vi "Wind_Turbine.vi"() -> (5 "Plug in titles":string[](array[string]), 7 "Plug in values":string[](array[string]))   [LabVIEW 2021]
uses:
  ADAM Client/Sub VIs/ADAM Controls/Channel_names.ctl
  <vilib>/Analysis/baseanly.llb/Mean (DBL).vi
  Globals/Meas_global.vi
  Globals/LDA_meas_global_1.vi
  <vilib>/Analysis/NI_AALBase.lvlib
  <vilib>/Analysis/NI_AALPro.lvlib
panel:
  in  "Time Shift":dbl
  out "X array":dbl[](array[numeric])
  out "WT Numbers":string[](array[string])
  out "WT Revolution Start times":dbl[](array[numeric])
  out "Laser Disp Index":i32
  out "Laser Phase lock index":i32
  out "Laser Status Index":i32
  out "L Status Phase lock index":i32
  in  "Tab Control":T1(tab)
  in  "Change Dem Voltages?":bool=TRUE
  in  "Allow large changes?":bool
  out "Turbine RPMs":cluster{i32[], "All WTs":dbl[]}(graph)
  out "All WTs":dbl[][](array[numeric]) format="%#.2g"
  out "Turbine Dem RPM":dbl[](array[numeric])
  out "Turbine Dem Voltage":dbl[](array[numeric])
  out "Cross Chs":cluster{dbl[], dbl[]}[](graph)
  in  "Cross_Corr to Phase Lock":i32[](listbox)
  in  "Channel to Phase lock":i32[](listbox)
  in  "Turbine to Phase Lock to":u16(ring) items=["RV (Ph)"]
  out "Inst Channels":cluster{dbl[], dbl[]}[](graph)
  in  "Add Phase data to results file":bool
  in  "Save Phase averaged Profiles":bool
  in  "Output Directory":path
  in  "Separation Character":string="\t"
  in  "Angular Step(deg)":dbl=1.0
  in  "Precision":string
  out "Av Disp 1":dbl
  out "Av Disp 2":dbl
  out "Av Disp 3":dbl
  out "Av Variance 1":dbl
  out "Av Variance 2":dbl
  out "Av Variance 3":dbl
  out "Angle 1":dbl format="%#_3g"
  out "Angle 2":dbl format="%#_3g"
  out "Angle 3":dbl format="%#_3g"
  out "Mean Blade 1":cluster{dbl, "Angular Step":dbl, dbl[]}(graph)
  out "slope 1":dbl format="%#_3g"
  out "Mean Blade 2":cluster{dbl, "Angular Step":dbl, dbl[]}(graph)
  out "Mean Blade 3":cluster{dbl, "Angular Step":dbl, dbl[]}(graph)
  out "slope 2":dbl format="%#_3g"
  out "slope 3":dbl format="%#_3g"
  out "Blade Positions":dbl[][](graph)
  out "Blade Angles":dbl[][](graph)
  out "Blade 1 Every Pass":dbl[](graph)
  out "Blade 2 Every Pass":dbl[](graph)
  out "Blade 3 Every Pass":dbl[](graph)
  out "Blade Analysis":string[][](table)
  in  "End Cut Deg":dbl
  in  "Start Cut Deg":dbl
  # "ADAM Channels"
  # "Rig_Name:Turbine_1:Dem_RPM"
  # "Rig_Name:Turbine_1:Dem_Volts"
  # "Mean RPM      SD RPM           Max-Min"
  # "Photo Darlington channel must have this symbol\nRV (Ph"
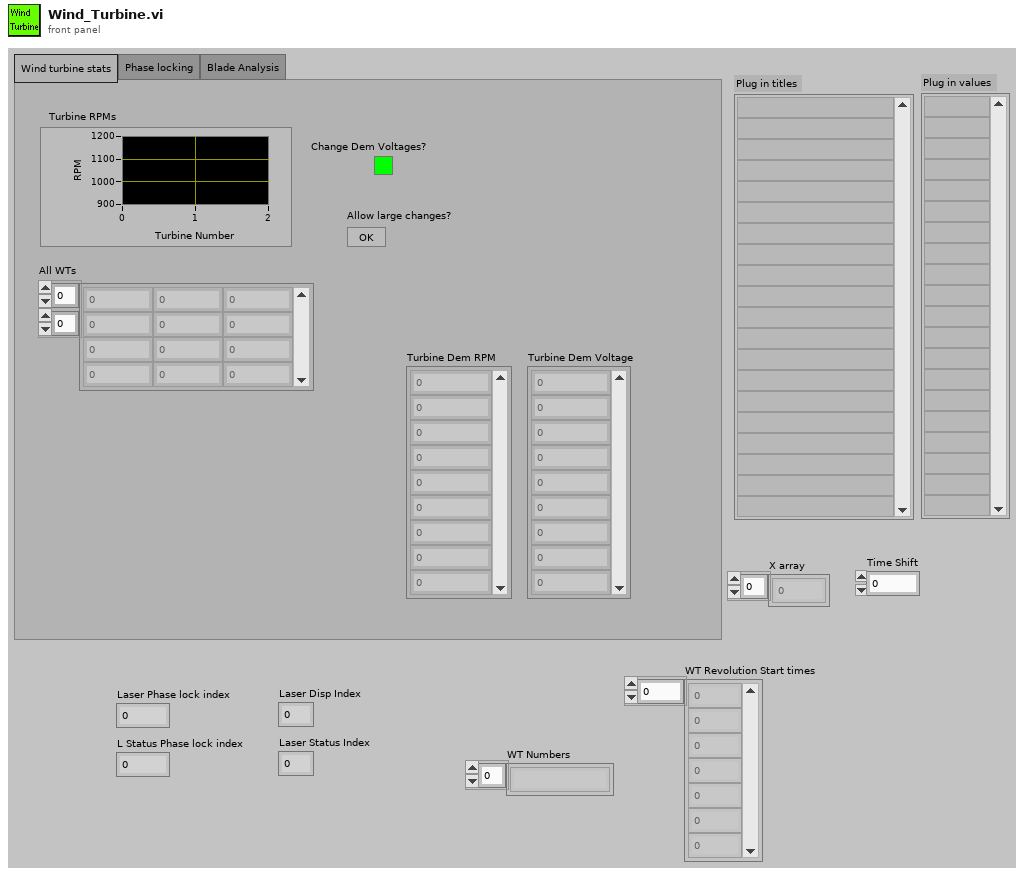
[diagram p1: front panel]
types:
  T1 = enum32{"Wind turbine stats", "Phase locking", "Blade Analysis"}
  T2 = typedef "Post_Process.ctl" = enum16{"Take New Data", "Post Process Raw Data File"}
  T3 = typedef "Analysis_info_cluster.ctl" = cluster{"Colour":u32, "Inst type":T4, "Inst name":string, "Symbol":string, "Code name":string, "Extra Info":string, "Inst Array":T5, "Extra Titles":string[], "Extra Values":string[], "U":dbl, "u^2":dbl, "u^3":dbl, "u^4":dbl, "Skew_u":dbl, "Kurt_u":dbl, "Sd Error in Mean":dbl, "% u'/U":dbl, "X":dbl, "Y":dbl, "Z":dbl, "Timescale integral Estimate":dbl, "Sd Error in Variance":dbl, "Calib File":path, "Calib Constants":dbl[], "Output Position":bool, "Stats":enum16{"None", "Basic", "Full"}, "Av Sampling Rate":dbl, "Av No of Samples":dbl, "Total Meas Time (s)":dbl, "ADAM Ch Name":string, "Max value":dbl, "Min value":dbl, "Req Sample Rate Hz":dbl, "Sync Delay Time (s)":dbl, "Ch No":i16, "Device":string, "Use Latest Calib":bool, "Port":string, "Metadata Ch Names":string[], "Metadata Ch Values":string[], "Label":string}
  T4 = typedef "Inst_type.ctl" = enum16{"Raw voltage", "Raw with zero offsetting", "Propeller anemometer", "Pressure Transducer", "Pitot-static tube", "Hot wire", "Cross wire 1", "Cross wire 2", "Generic Linear", "Generic Polynomial", "Generic BackPoly", "Fast FID", "Thermocouple", "Cold wire", "Pulsed Wire", "LDA Vel", "LDA Tran time", "LDA Arr time", "Microphone"}
  T5 = typedef "Instrument_Array.ctl" = enum16{"PWA", "LDA", "Analogue"}
  T6 = typedef "Time_Trace_Cluster.ctl" = cluster{"Weighting":dbl[], "Voltage":dbl[], "Eng Values":dbl[]}
  T7 = typedef "Channel_names.ctl" = enum16{"Active Only", "Active + Off", "All Channels", "Changeable Only"}
  T8 = typedef "Shift_Cluster.ctl" = cluster{"Stats":dbl[], "Spectra_Auto":dbl[], "Histogram":dbl[], "Hist Max":dbl, "Hist Min":dbl, "No of Samples":i32, "No in plume":i32, "Weight sum":dbl, "No Of Hist bins":i32, "TimeTrace Max":dbl, "Time Trace Min":dbl, "Trace St Deviation":dbl}
  T9 = typedef "Cross_Moments_Shift_Cluster.ctl" = cluster{"Stats":dbl[], "Resampled No of Samples":i32, "Resampled delta T":dbl, "Cross Correlation":dbl[]}
  T10 = cluster{"X array":dbl[], "Phase locked uw/u'w'":dbl[]}
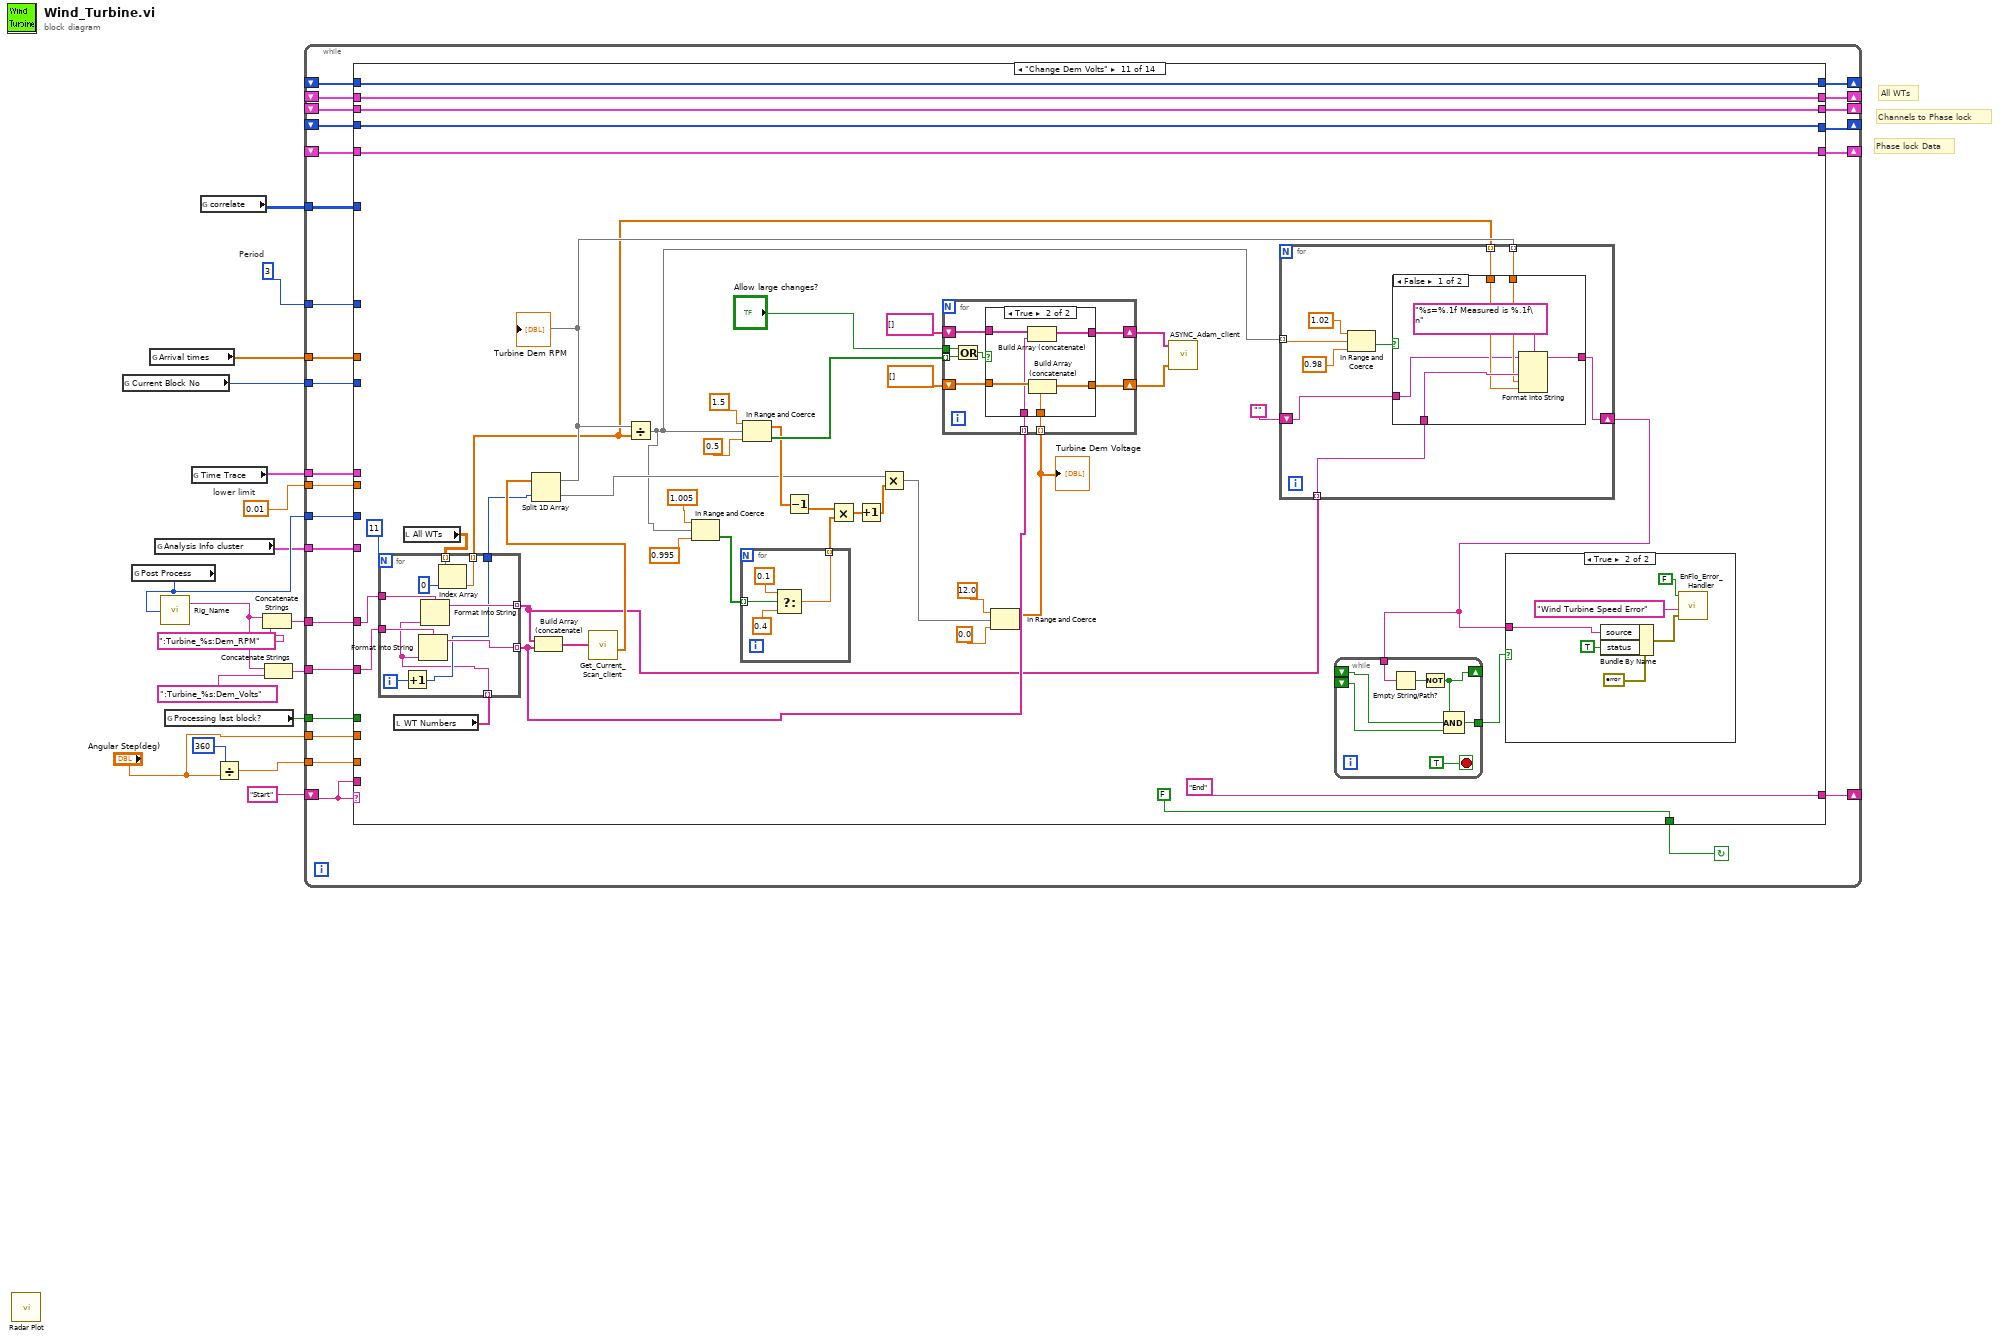
[diagram p0: block diagram]
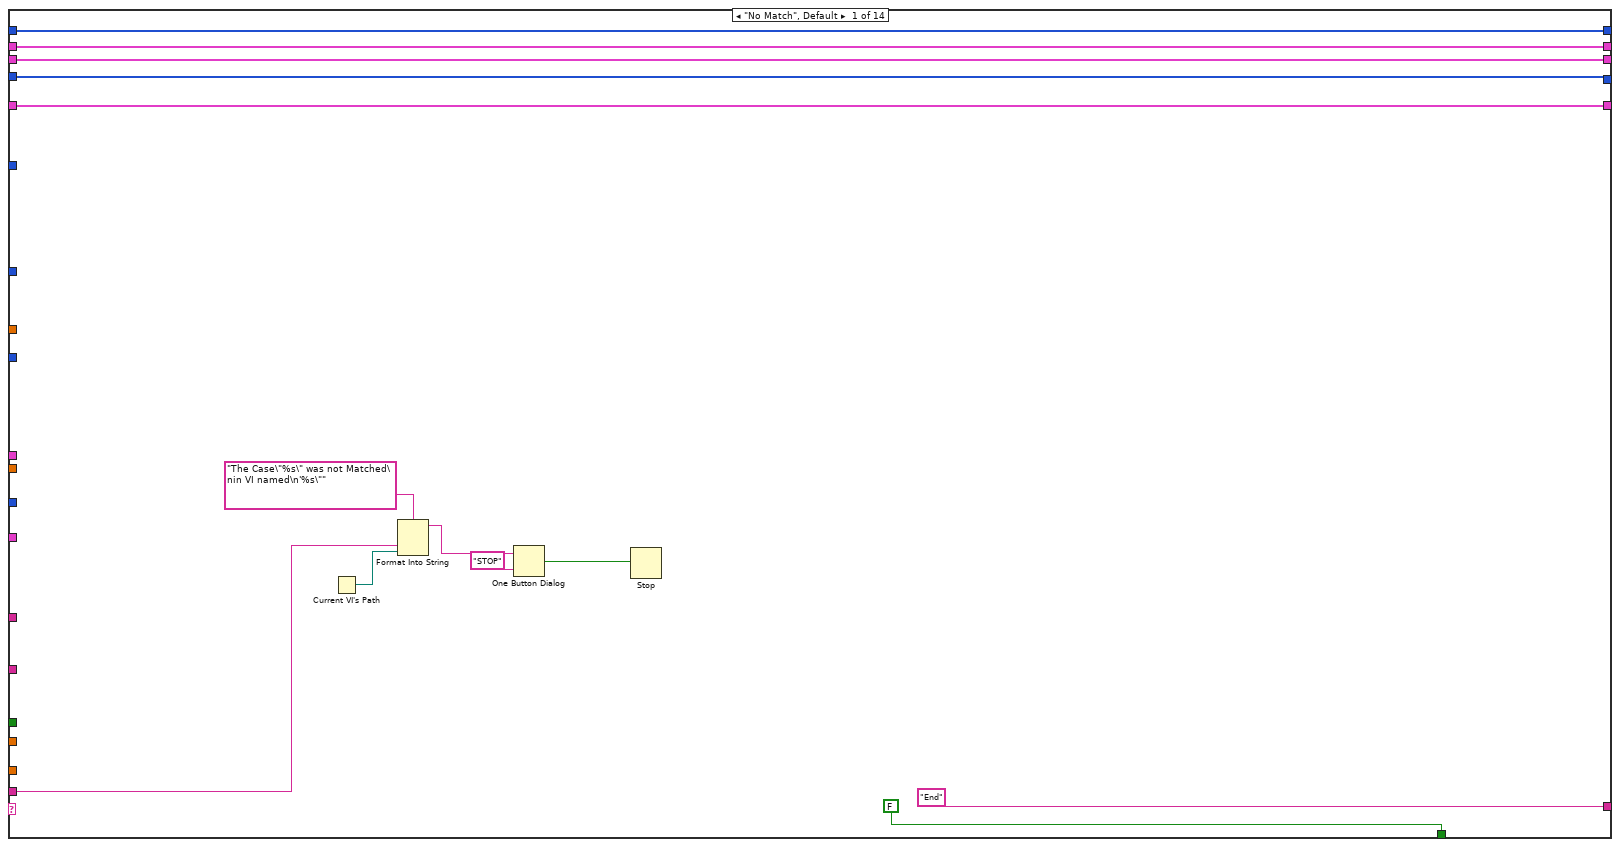
[diagram p2: hidden frame]
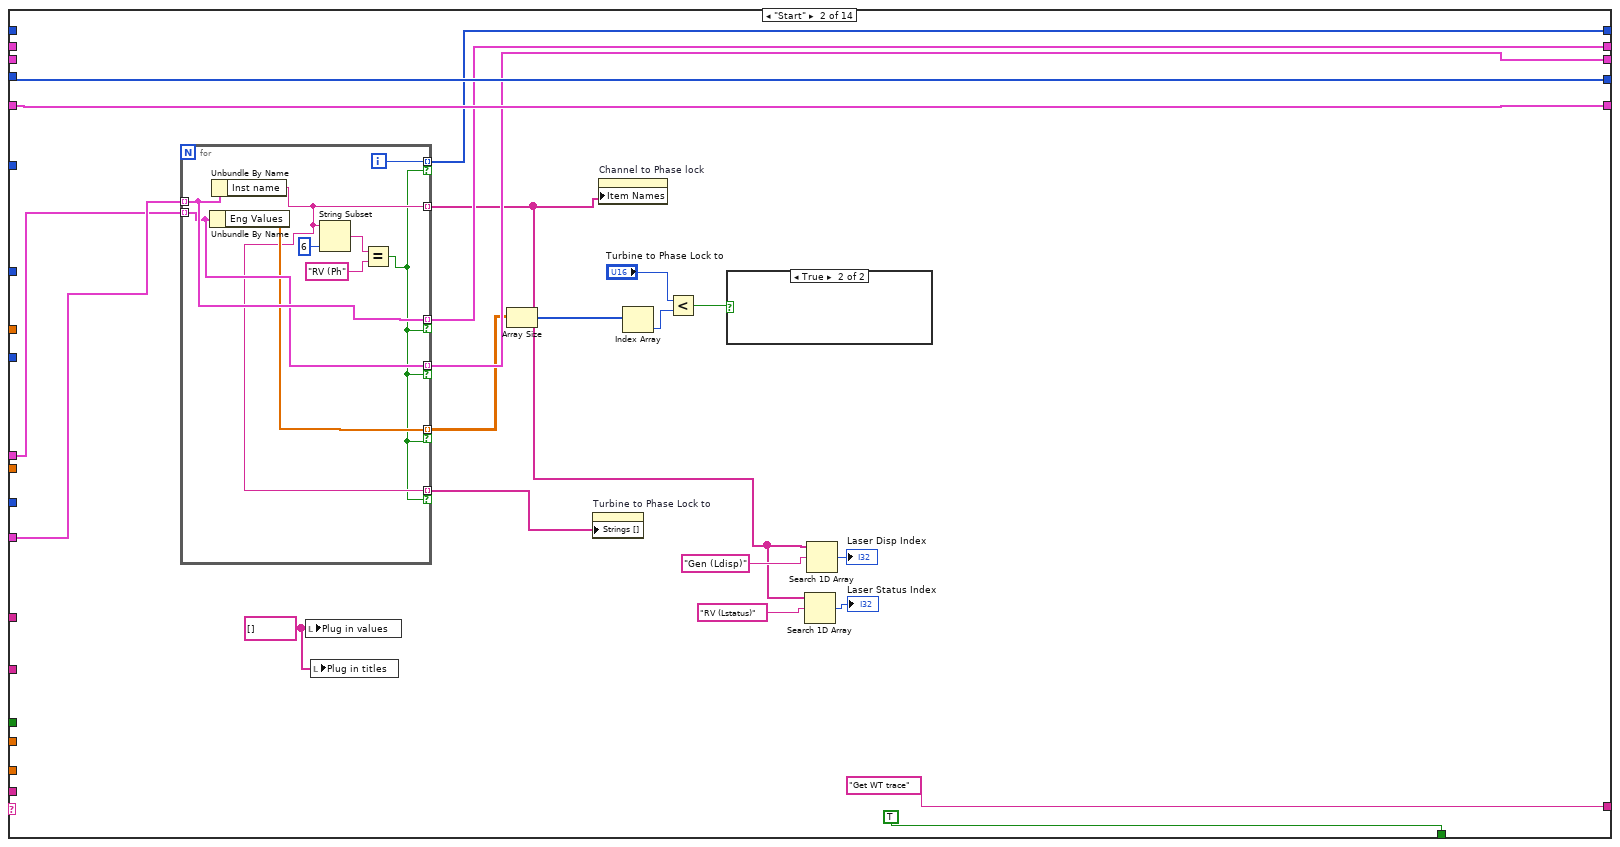
[diagram p3: hidden frame]
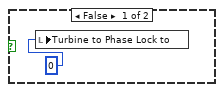
[diagram p4: hidden frame]
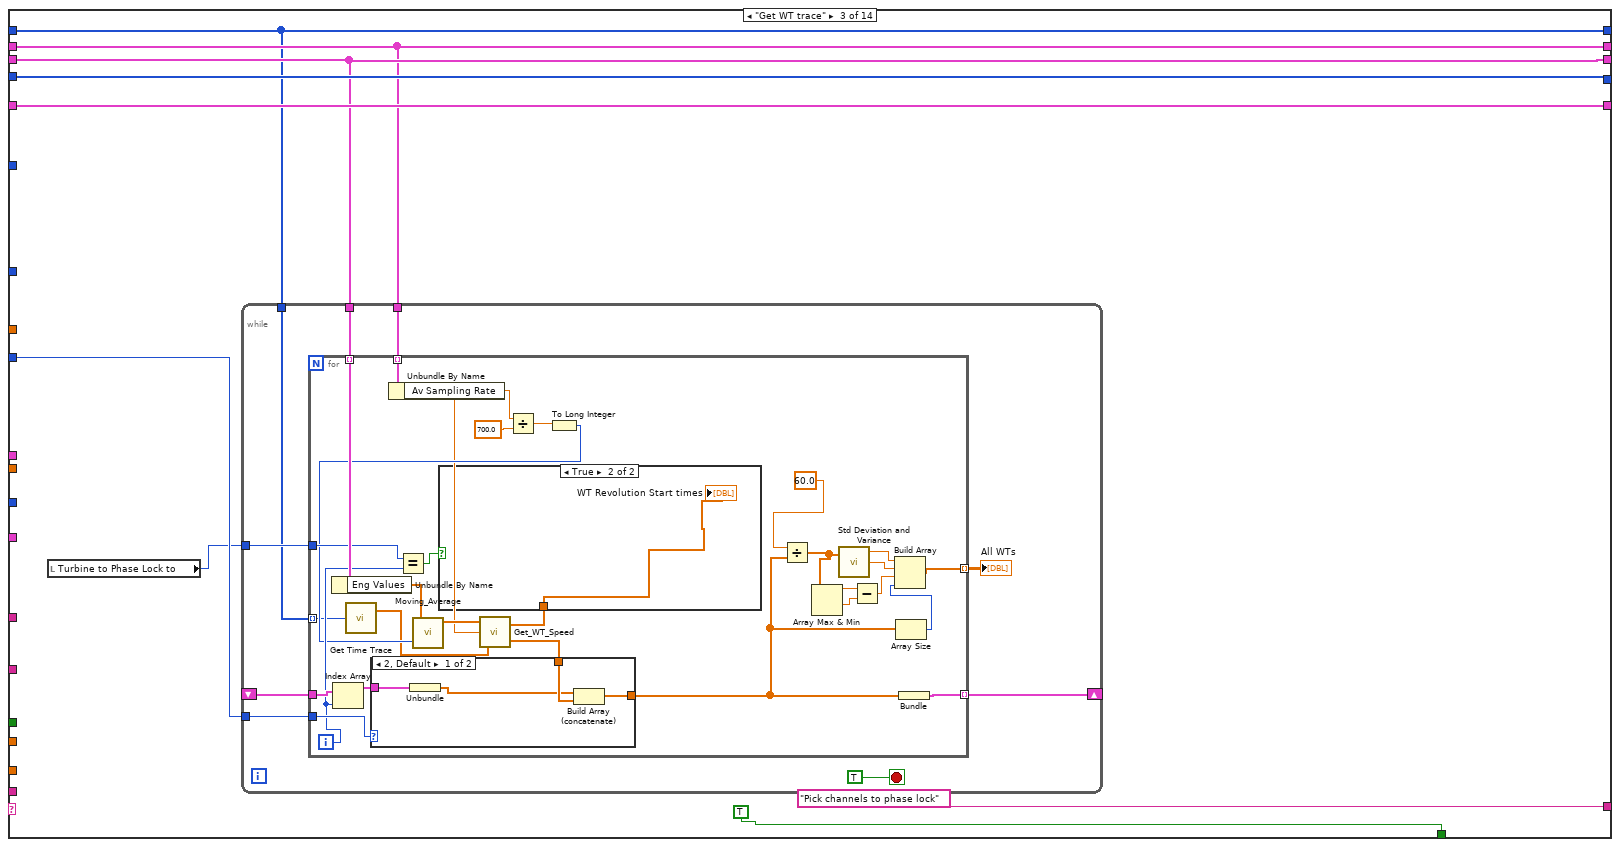
[diagram p5: hidden frame]
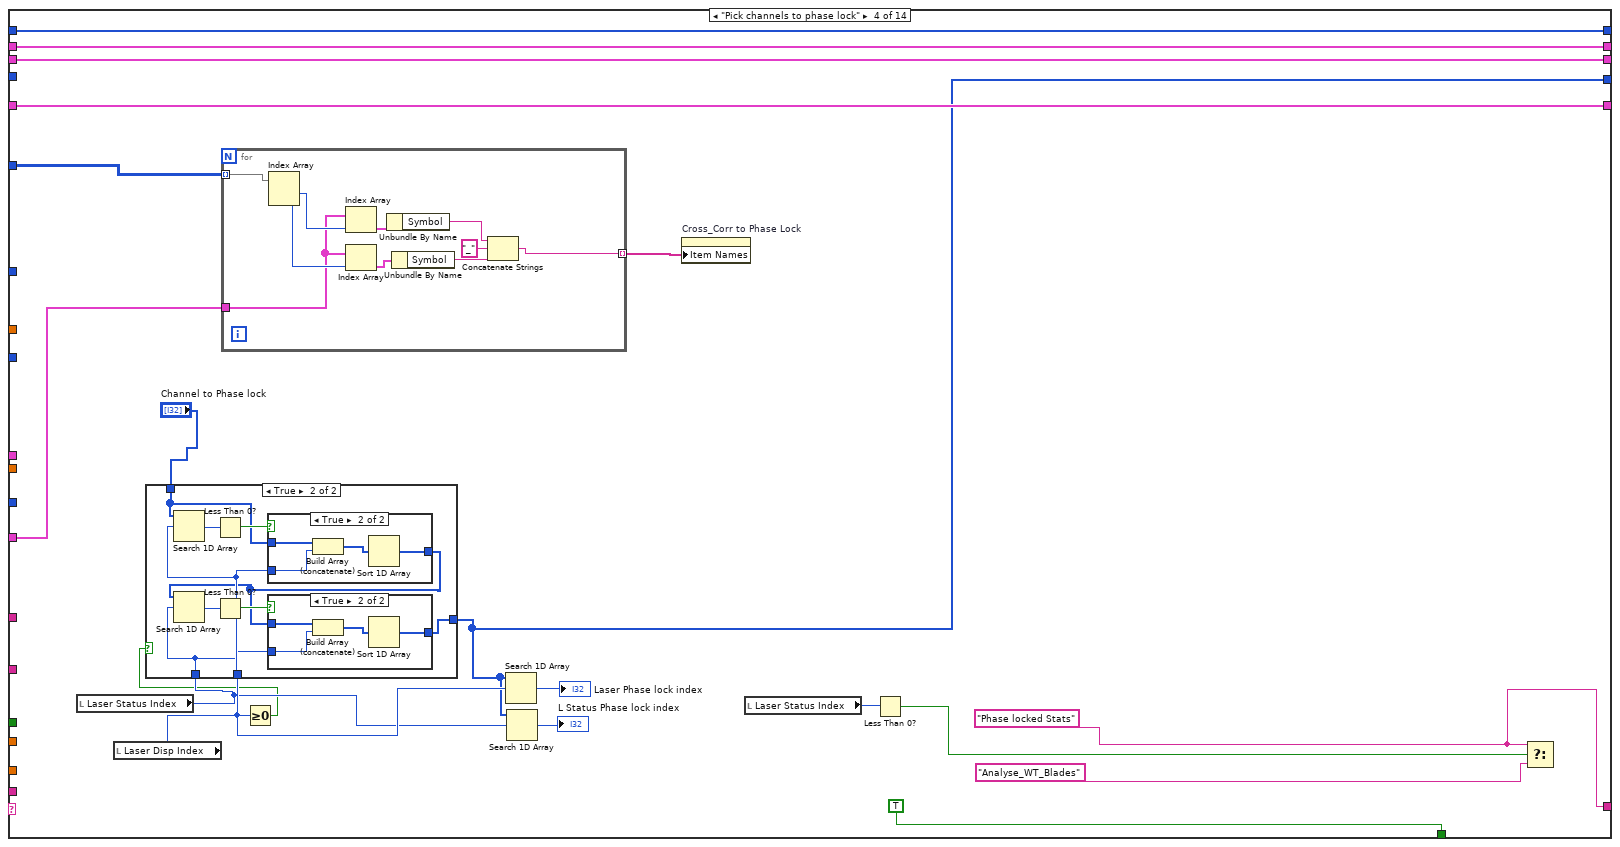
[diagram p8: hidden frame]
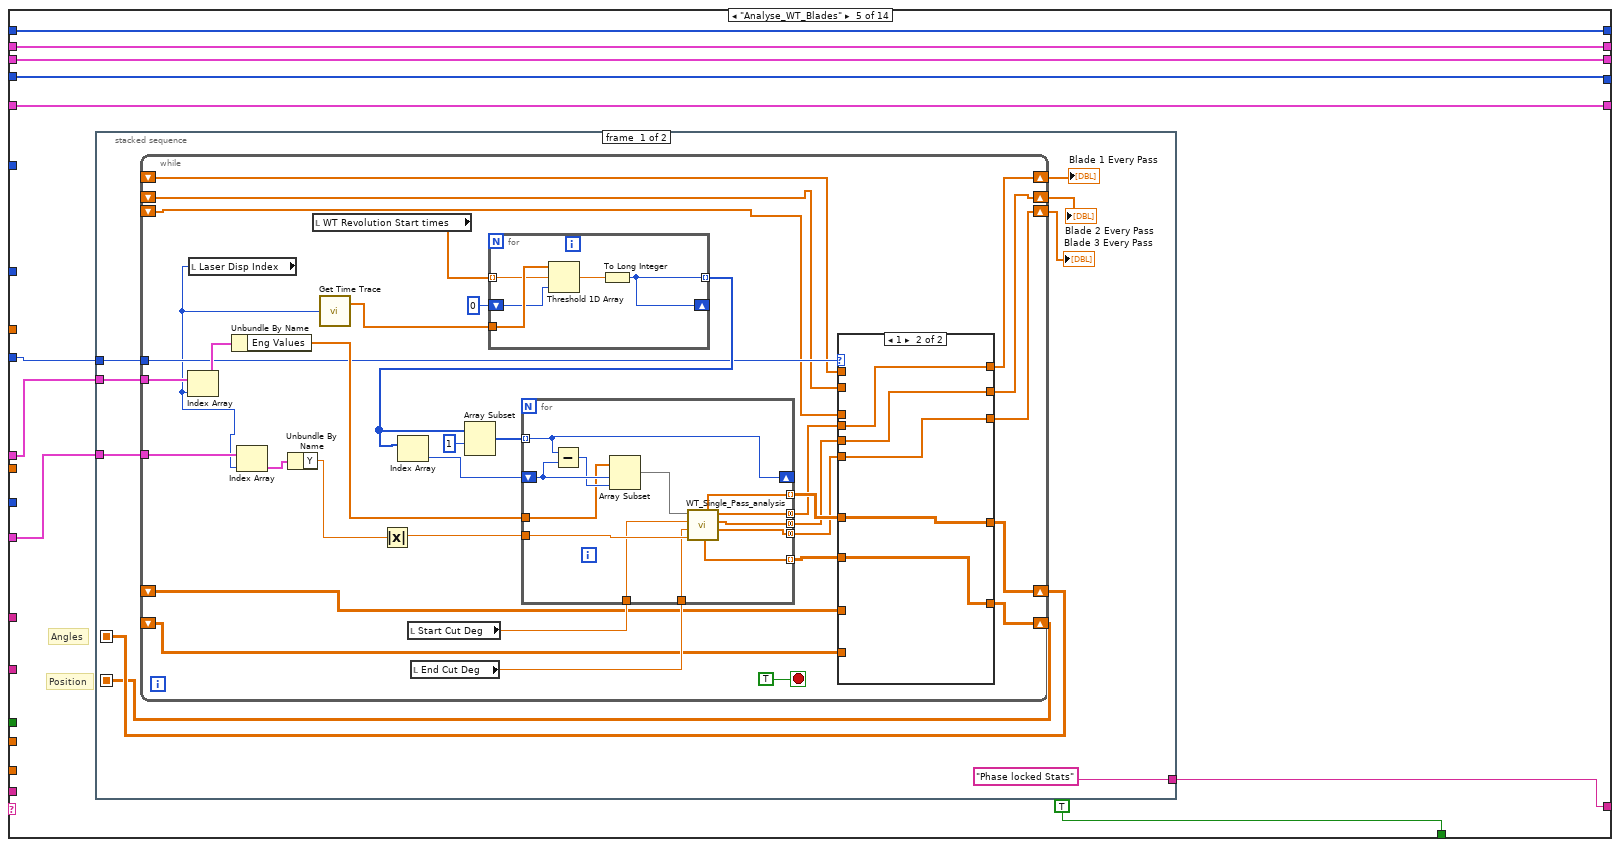
[diagram p12: hidden frame]
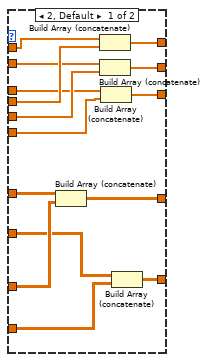
[diagram p13: hidden frame]
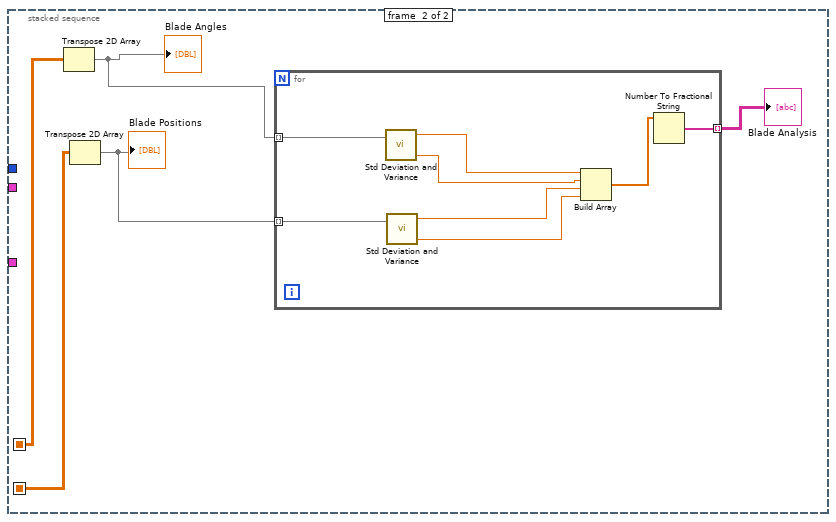
[diagram p14: hidden frame]
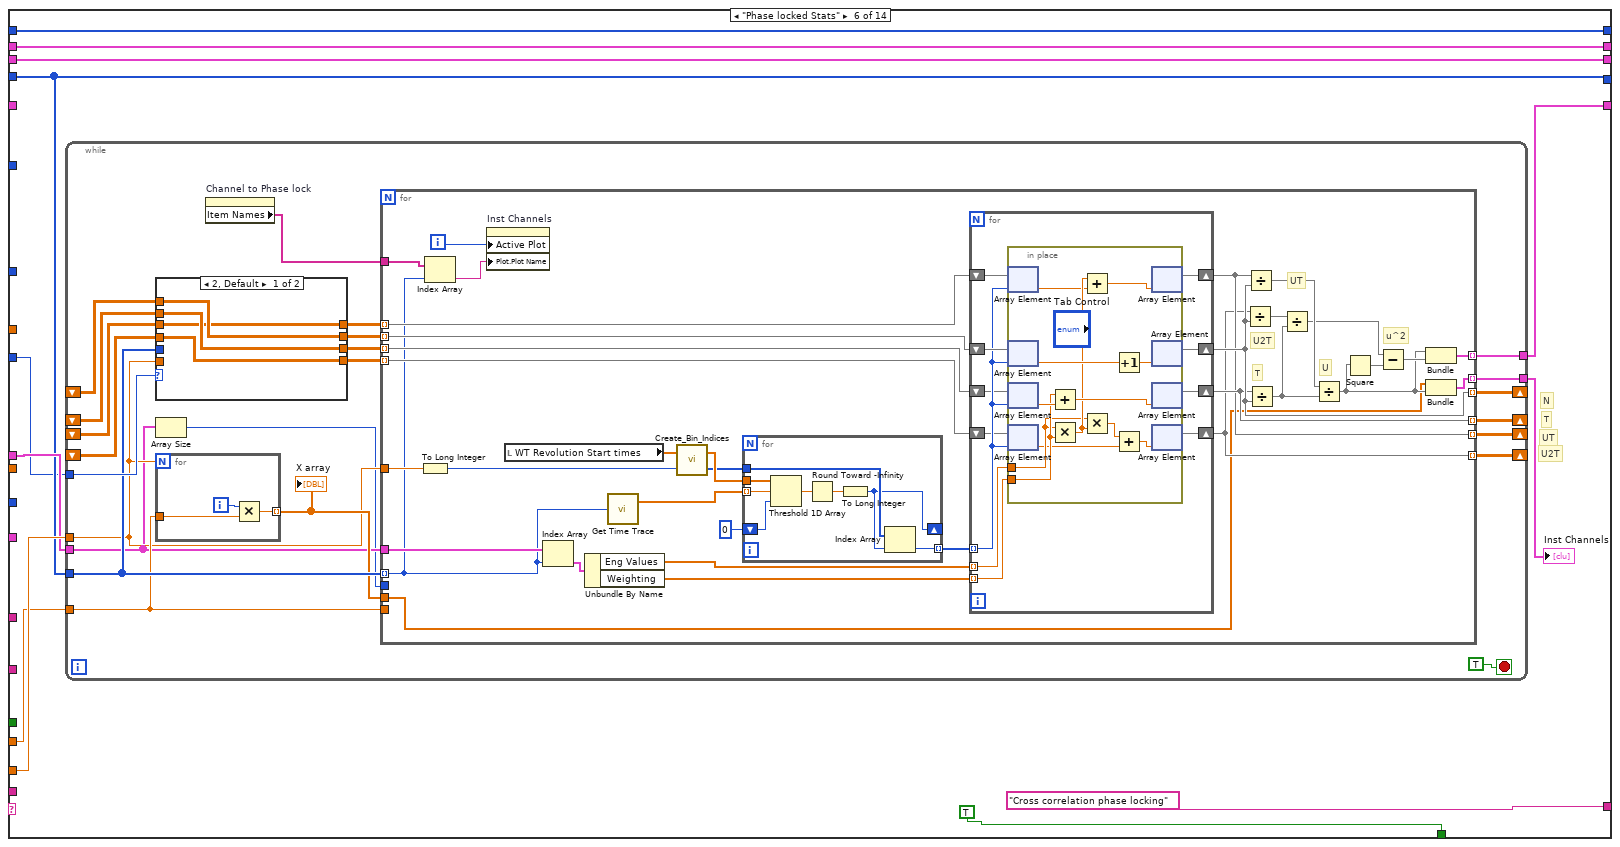
[diagram p15: hidden frame]
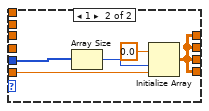
[diagram p16: hidden frame]
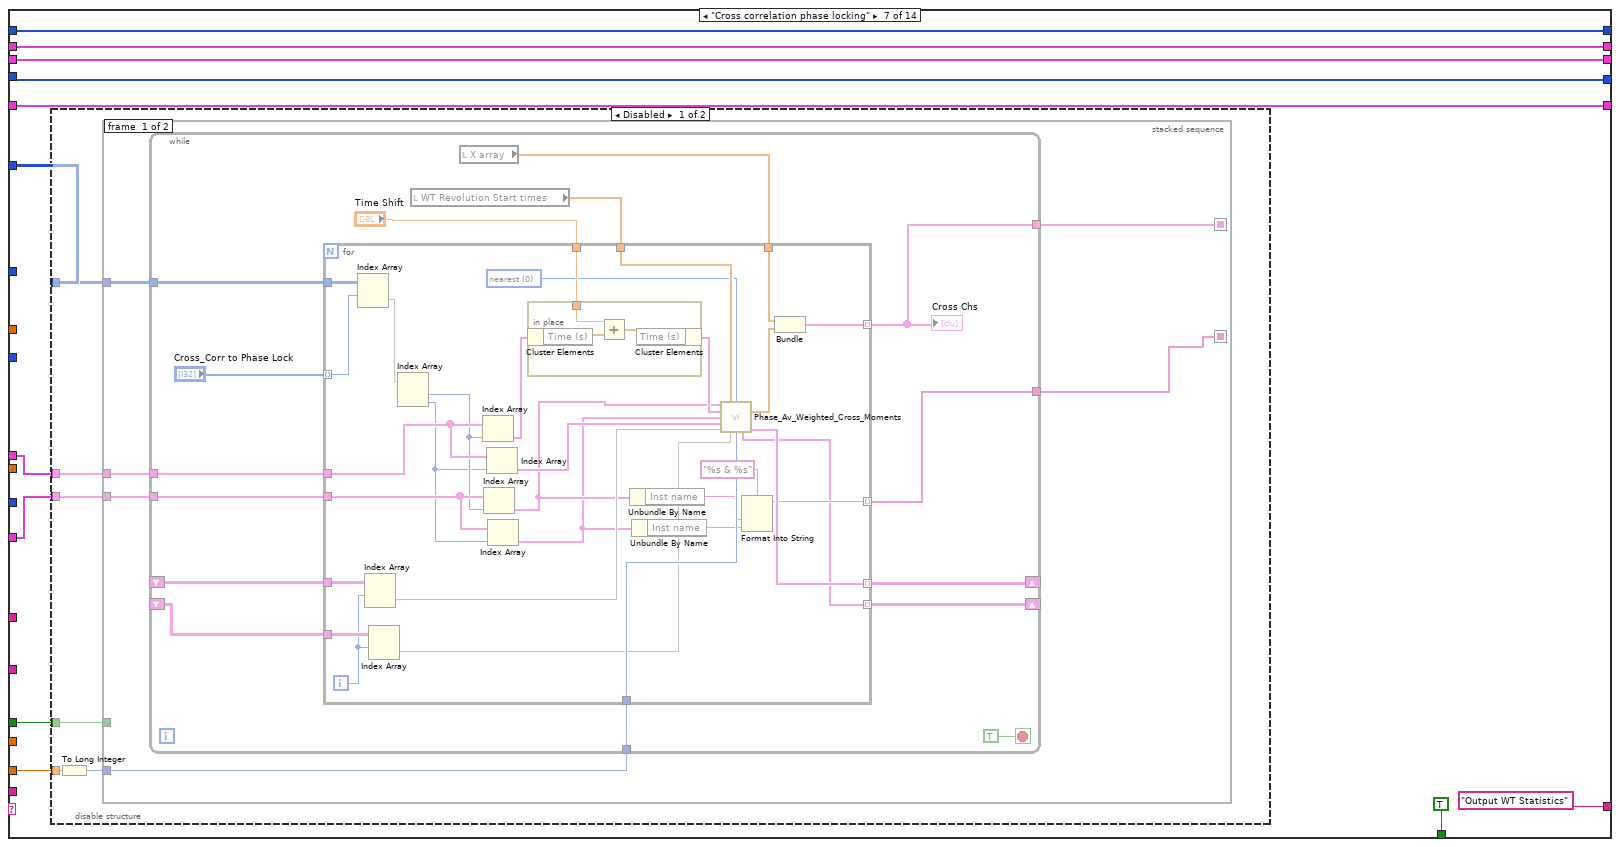
[diagram p17: hidden frame]
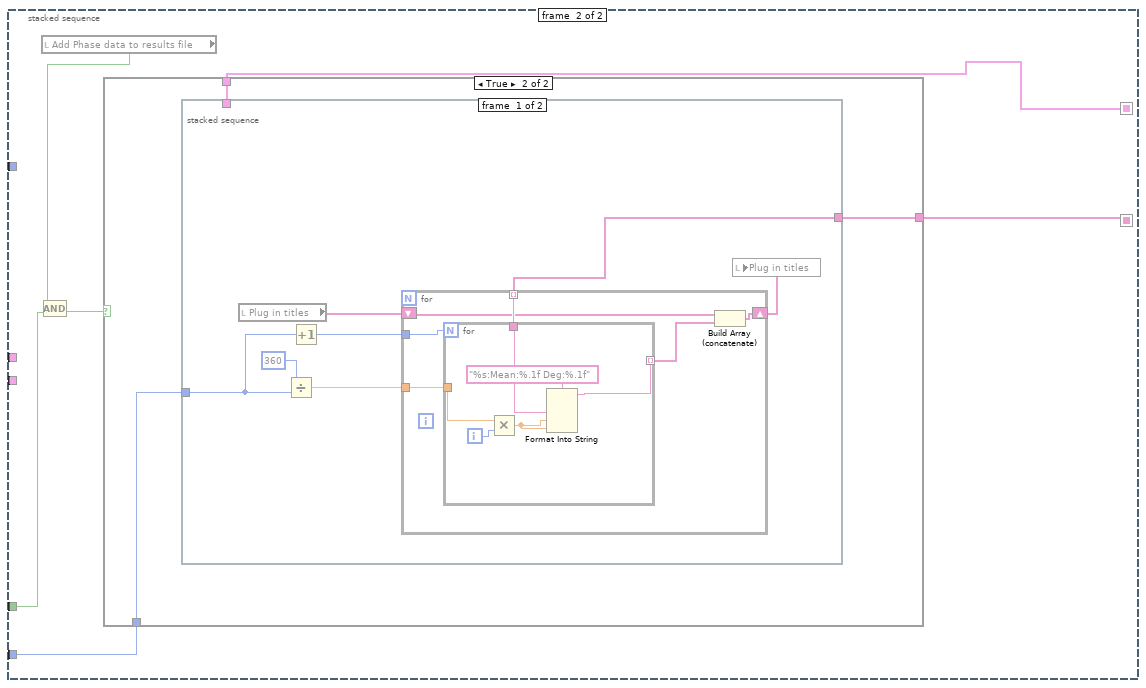
[diagram p18: hidden frame]
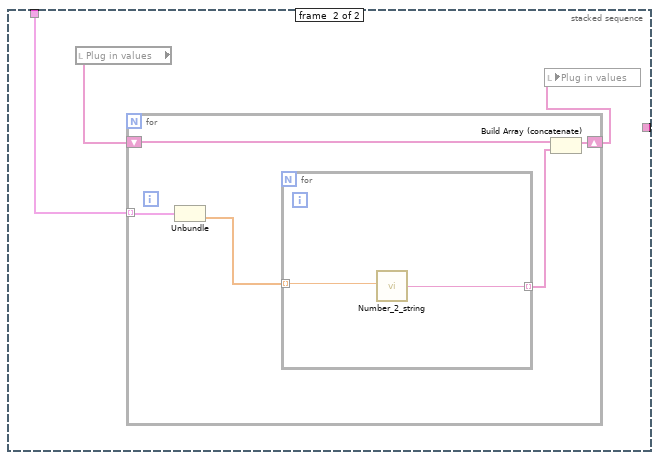
[diagram p20: hidden frame]
diagram:
  w17 = 3  # Period
  w18 = 0.01  # lower limit
  # "Phase lock Data"
  # "Channels to Phase lock"
  # "All WTs"
  n1 = call <vilib>:"Radar Plot.vi"() -> ()  [unwired: 15 in, 1 out]
  n2 = global read "Meas_global.vi" "Current Block No"() -> (w5:i32)
  n3 = global read "Meas_global.vi" "Post Process"() -> (w16:T2)
  n4 = global read "LDA_meas_global_1.vi" "Arrival times"() -> (w8:dbl[])
  n5 = global read "Meas_global.vi" "Analysis Info cluster"() -> (w7:T3[])
  n6 = call "Rig_Name.vi"("Post Process"=w16) -> ("Rig Setup before dash"=w13:string)  [unwired: 1 out]
  n7 = global read "Meas_global.vi" "Processing last block?"() -> (w10:bool)
  n8 = global read "Meas_global.vi" "Time Trace"() -> (w3:T6[])
  n9 = global read "Meas_global.vi" "correlate"() -> (w1:i32[][])
  n10 = Divide(x=360, y="Angular Step(deg)") -> (x/y=w6:dbl)
  n11 = Concatenate Strings(w13, ":Turbine_%s:Dem_RPM") -> (w12:string)
  n12 = Concatenate Strings(w13, ":Turbine_%s:Dem_Volts") -> (w15:string)
  n13 = while {
    tunnel: w5 -> [w44]
    tunnel: w15 -> [w43]
    tunnel: w12 -> [w42]
    tunnel: w18 -> [w41]
    tunnel: w17 -> [w40]
    tunnel: w16 -> [w39]
    tunnel: w7 -> [w38]
    shift-right: [w22] -> _
    shift-left: "Start" -> [w36]
    tunnel: w10 -> [w35]
    tunnel: w6 -> [w34]
    tunnel: w8 -> [w33]
    tunnel: "Angular Step(deg)" -> [w32]
    shift-right: [w31] -> _
    shift-left: _ -> [w30]
    shift-right: [w28] -> _
    shift-left: _ -> [w29]
    shift-right: [w27] -> _
    shift-left: _ -> [w26]
    tunnel: w3 -> [w25]
    shift-right: [w24] -> _
    shift-left: _ -> [w23]
    tunnel: w1 -> [w21]
    shift-right: [w20] -> _
    shift-left: _ -> [w19]
    stop <- w37 continue-if-true
    n14 = case shown="\"Change Dem Volts\"" w36 {
      tunnel: w44 -> [_ _ w95 _ w193 w299 _ _ _ _ _ _ _ _]
      tunnel: w43 -> [_ _ _ _ _ _ _ _ _ w829 w907 _ _ _]
      tunnel: w42 -> [_ _ _ _ _ _ _ _ _ w830 w888 _ _ _]
      tunnel: w41 -> [_ _ _ _ _ _ _ _ _ _ _ _ _ _]
      tunnel: w40 -> [_ _ _ _ _ _ _ _ _ _ _ _ _ _]
      tunnel: w39 -> [_ _ _ _ _ _ _ _ _ w838 _ _ _ _]
      tunnel: w38 -> [_ w78 _ w146 w195 _ w410 _ w592 _ _ _ _ _]
      tunnel: ["End" "Get WT trace" "Pick channels to phase lock" w143 w192 "Cross correlation phase locking" "Output WT Statistics" w542 w597 w837 "End" ("f") "Check Folder Name" "Save Phase locked data" "End"] -> w22
      tunnel: [FALSE ("Change Control Voltage?") TRUE ("Processing last block?") TRUE TRUE ("Change Control Voltage?") TRUE ("Change Control Voltage?") TRUE TRUE ("Change Control Voltage?") TRUE ("Change Control Voltage?") w598 w836 FALSE ("Change Control Voltage?") w977 w1029 FALSE ("Change Control Voltage?")] -> w37
      tunnel: w36 -> [w52 _ _ _ _ _ _ _ _ _ _ _ _ _]
      tunnel: w35 -> [_ _ _ _ _ _ w408 _ w599 w835 _ w975 _ _]
      tunnel: w34 -> [_ _ _ _ _ w306 w409 _ w601 _ _ w973 _ _]
      tunnel: w33 -> [_ _ _ _ _ _ _ _ _ _ _ _ _ _]
      tunnel: w32 -> [_ _ _ _ _ w305 _ _ w600 _ _ _ _ w1047]
      tunnel: [w49 w64 w90 w160 w200 w304 w416 w539 w596 w834 w887 w972 w1027 w1050] -> w31
      tunnel: w30 -> [w49 _ w90 w160 w200 w304 w416 w539 w596 w834 w887 w972 w1027 w1050]
      tunnel: w29 -> [w48 w65 w93 _ w198 w300 w414 w538 w595 w833 w886 w971 w1026 w1049]
      tunnel: [w48 w65 w93 w151 w198 w300 w414 w538 w595 w833 w886 w971 w1026 w1049] -> w28
      tunnel: [w47 w66 w92 w155 w197 w298 w413 w537 w593 w832 w885 w969 w1025 w1048] -> w27
      tunnel: w26 -> [w47 w66 w92 w155 w197 _ w413 w537 w593 w832 w885 w969 w1025 w1048]
      tunnel: w25 -> [_ w67 _ _ w196 w301 w411 _ _ _ _ _ _ _]
      tunnel: [w46 w63 w91 w154 w199 w302 w415 w536 w594 w831 w884 w970 w1024 w1046] -> w24
      tunnel: w23 -> [w46 _ w91 w154 w199 w302 w415 w536 w594 w831 w884 w970 w1024 w1046]
      tunnel: w21 -> [_ _ _ w144 _ _ w412 _ _ _ _ _ _ _]
      tunnel: [w45 w58 w89 w142 w191 w295 w407 w517 w591 w828 w869 w968 w1023 w1045] -> w20
      tunnel: w19 -> [w45 _ w89 w142 w191 w295 w407 w517 w591 w828 w869 w968 w1023 w1045]
      frame "No Match", Default {
        n15 = Current VI's Path() -> (path=w53:path)
        n16 = Format Into String(format string="The Case\"%s\" was not Matched\nin VI named\n'%s\"" ("Format String"), w52, w53) -> (resulting string=w56:string)  [unwired: 2 in, 1 out]
        n17 = One Button Dialog(message=w56, button name ("OK")="STOP") -> (true=w54:bool)
        n18 = Stop(stop? (T)=w54) -> ()
      }
      frame "Start" {
        w59 = string[] [] ("Plug in values")
        n19 = for {
          tunnel: w78 -> [w85] mode=indexing
          tunnel: [w82] -> w60 mode=indexing
          tunnel: w67 -> [w84] mode=indexing
          tunnel: [w85] -> w64 mode=indexing if=w80
          tunnel: [w84] -> w63 mode=indexing if=w80
          tunnel: [w83] -> w62 mode=indexing if=w80
          tunnel: [w82] -> w61 mode=indexing if=w80
          tunnel: [w81] -> w58 mode=indexing if=w80
          i -> [w81]
          n20 = Unbundle By Name(w84) -> ("Eng Values"=w83:dbl[])
          n21 = Unbundle By Name(w85) -> ("Inst name"=w82:string)
          n22 = String Subset(string=w82, length (rest)=6 ("length (rest)")) -> (substring=w86:string)  [unwired: 1 out]
          n23 = Equal?(x=w86, y="RV (Ph") -> (x = y?=w80:bool)
        }
        n24 = local write "Plug in values"(w59) -> ()
        n25 = local write "Plug in titles"(w59) -> ()
        n26 = Array Size(array=w62) -> (size(s)=w69:i32[])
        n27 = property on="Turbine to Phase Lock to" class="Ring (strict)"("Strings []"=w61) -> ()  [unwired: 2 in, 2 out]
        n28 = property on="Channel to Phase lock" class="LstBox (strict)"("Item Names"=w60) -> ()  [unwired: 2 in, 2 out]
        n29 = Index Array(array=w69) -> (element=w68:i32)  [unwired: 1 in]
        n30 = Less?(x="Turbine to Phase Lock to", y=w68) -> (x < y?=w74:bool)
        n31 = case shown="True" w74 {
          frame False {
            n32 = local write "Turbine to Phase Lock to"(0) -> ()
          }
          frame True {
          }
        }
        n33 = Search 1D Array(1D array=w60, element="RV (Lstatus)") -> (index of element=→"Laser Status Index":i32)  [unwired: 1 in]
        n34 = Search 1D Array(1D array=w60, element="Gen (Ldisp)") -> (index of element=→"Laser Disp Index":i32)  [unwired: 1 in]
      }
      frame "Get WT trace" {
        n35 = local read "Turbine to Phase Lock to"() -> (w94:u16)
        n36 = while {
          tunnel: w95 -> [w106]
          shift-right: [w102] -> _
          shift-left: _ -> [w105]
          tunnel: w91 -> [w101]
          tunnel: w94 -> [w100]
          tunnel: w90 -> [w99]
          tunnel: w89 -> [w98]
          stop <- TRUE stop-if-true
          n37 = for {
            tunnel: w106 -> [w134]
            tunnel: w105 -> [w126]
            tunnel: [w127] -> w103 mode=indexing
            tunnel: [w123] -> w102 mode=indexing
            tunnel: w101 -> [w122] mode=indexing
            tunnel: w100 -> [w119]
            tunnel: w99 -> [w117] mode=indexing
            tunnel: w98 -> [w108] mode=indexing
            i -> [w120]
            n38 = Unbundle By Name(w122) -> ("Eng Values"=w121:dbl[])
            n39 = Index Array(array=w126, index=w120) -> (element=w125:cluster{"Time per Cycle":dbl[]})
            n40 = call "Get Time Trace.vi"("Channel Index"=w108) -> ("Time (s)"=w107:dbl[])  [unwired: 1 out]
            n41 = Unbundle By Name(w117) -> ("Av Sampling Rate"=w113:dbl)
            n42 = Equal?(x=w119, y=w120) -> (x = y?=w118:bool)
            n43 = Divide(x=w113, y=700.0) -> (x/y=w116:dbl)
            n44 = To Long Integer(number=w116) -> (32bit integer=w114:i32)
            n45 = call "Moving_Average.vi"("Period"=w114, "Input Array"=w121) -> ("N+1-Period"=w135:dbl[])
            n46 = call "Get_WT_Speed.vi"("Time (s)"=w107, "Av Sampling Rate"=w113, "Opto Trace"=w135) -> ("Time per Cycle"=w133:dbl[], "Start Cycle Time"=w112:dbl[])
            n47 = case shown="2, Default" w134 {
              tunnel: [w139 w141] -> w111
              tunnel: w133 -> [w140 w141]
              tunnel: w125 -> [w138 _]
              frame 2, Default {
                n48 = Unbundle(w138) -> ("Time per Cycle"=w137:dbl[])
                n49 = Build Array (concatenate)(w137, w140) -> (w139:dbl[])
              }
              frame 1 {
              }
            }
            n50 = case shown="True" w118 {
              tunnel: w112 -> [_ w136]
              frame False {
              }
              frame True {
                "WT Revolution Start times" <- w136
              }
            }
            n51 = Divide(x=60.0, y=w111) -> (x/y=w109:dbl[])
            n52 = Array Max & Min(array=w109) -> (max value=w132:dbl, min value=w131:dbl)  [unwired: 2 out]
            n53 = call <vilib>:"Std Deviation and Variance.vi"("X"=w109) -> ("mean"=w130:dbl, "standard deviation"=w129:dbl)  [unwired: 1 in, 1 out]
            n54 = Subtract(x=w132, y=w131) -> (x-y=w128:dbl)
            n55 = Array Size(array=w111) -> (size(s)=w124:i32)
            n56 = Build Array(w130, w129, w128, w124) -> (w127:dbl[])
            n57 = Bundle("Time per Cycle"=w111) -> (w123:cluster{"Time per Cycle":dbl[]})  [unwired: 1 in]
          }
          "All WTs" <- w103
        }
      }
      frame "Pick channels to phase lock" {
        w143 = "Phase locked Stats" ("f")
        n58 = local read "Laser Status Index"() -> (w157:i32)
        n59 = local read "Laser Disp Index"() -> (w158:i32)
        n60 = for {
          tunnel: w144 -> [w170] mode=indexing
          tunnel: w146 -> [w167]
          tunnel: [w161] -> w145 mode=indexing
          n61 = Index Array(array=w170) -> (element #1=w169:i32, element #2=w168:i32)  [unwired: 2 in]
          n62 = Index Array(array=w167, index=w169) -> (element=w166:T3)
          n63 = Index Array(array=w167, index=w168) -> (element=w165:T3)
          n64 = Unbundle By Name(w166) -> ("Symbol"=w164:string)
          n65 = Unbundle By Name(w165) -> ("Symbol"=w163:string)
          n66 = Concatenate Strings(w164, "_" ("string"), w163) -> (w161:string)
        }
        n67 = Greater Or Equal To 0?(x=w158) -> (x >= 0?=w156:bool)
        n68 = case shown="True" w156 {
          tunnel: "Channel to Phase lock" -> [w171 w178]
          tunnel: w158 -> [_ w177]
          tunnel: [w171 w174] -> w151
          tunnel: w157 -> [_ w172]
          frame False {
          }
          frame True {
            n69 = Search 1D Array(1D array=w178, element=w177) -> (index of element=w180:i32)  [unwired: 1 in]
            n70 = Less Than 0?(x=w180) -> (x < 0?=w179:bool)
            n71 = case shown="True" w179 {
              tunnel: w178 -> [w186 w190]
              tunnel: w177 -> [_ w189]
              tunnel: [w186 w187] -> w173
              frame False {
              }
              frame True {
                n72 = Build Array (concatenate)(w190, w189) -> (w188:i32[])
                n73 = Sort 1D Array(array=w188) -> (sorted array=w187:i32[])
              }
            }
            n74 = Search 1D Array(1D array=w173, element=w172) -> (index of element=w175:i32)  [unwired: 1 in]
            n75 = Less Than 0?(x=w175) -> (x < 0?=w176:bool)
            n76 = case shown="True" w176 {
              tunnel: w173 -> [w181 w185]
              tunnel: w172 -> [_ w184]
              tunnel: [w181 w182] -> w174
              frame False {
              }
              frame True {
                n77 = Build Array (concatenate)(w185, w184) -> (w183:i32[])
                n78 = Sort 1D Array(array=w183) -> (sorted array=w182:i32[])
              }
            }
          }
        }
        n79 = Search 1D Array(1D array=w151, element=w158) -> (index of element=→"Laser Phase lock index":i32)  [unwired: 1 in]
        n80 = Search 1D Array(1D array=w151, element=w157) -> (index of element=→"L Status Phase lock index":i32)  [unwired: 1 in]
        n81 = property on="Cross_Corr to Phase Lock" class="LstBox (strict)"("Item Names"=w145) -> ()  [unwired: 2 in, 2 out]
        n82 = local read "Laser Status Index"() -> (w149:i32)
        n83 = Less Than 0?(x=w149) -> (x < 0?=w148:bool)
        n84 = Select(t=w143, s=w148, f="Analyse_WT_Blades") -> ()  [unwired: 1 out]
      }
      frame "Analyse_WT_Blades" {
        # "Position"
        # "Angles"
        n85 = stacked-sequence {
          seq-local: [w204 _] -> [_ w285]
          seq-local: [w205 _] -> [_ w286]
          tunnel: w196 -> [w209 _]
          tunnel: w195 -> [w208 _]
          tunnel: w193 -> [w207 _]
          tunnel: ["Phase locked Stats" ("f") _] -> w192
          frame #0 {
            n86 = while {
              tunnel: w209 -> [w243]
              tunnel: w208 -> [w234]
              shift-right: [w224] -> w205
              shift-left: _ -> [w225]
              shift-right: [w221] -> w204
              shift-left: _ -> [w222]
              tunnel: w207 -> [w227]
              shift-right: [w219] -> w203
              shift-left: _ -> [w218]
              shift-right: [w214] -> w202
              shift-left: _ -> [w215]
              shift-right: [w212] -> w201
              shift-left: _ -> [w213]
              stop <- TRUE stop-if-true
              n87 = local read "Laser Disp Index"() -> (w211:i32)
              n88 = Index Array(array=w243, index=w211) -> (element=w242:T6)
              n89 = Unbundle By Name(w242) -> ("Eng Values"=w235:dbl[])
              n90 = Index Array(array=w234, index=w211) -> (element=w233:T3)
              n91 = Unbundle By Name(w233) -> ("Y"=w232:dbl)
              n92 = local read "WT Revolution Start times"() -> (w241:dbl[])
              n93 = call "Get Time Trace.vi"("Channel Index"=w211) -> ("Time (s)"=w210:dbl[])  [unwired: 1 out]
              n94 = Absolute Value(x=w232) -> (abs(x)=w231:dbl)
              n95 = local read "Start Cut Deg"() -> (w230:dbl)
              n96 = local read "End Cut Deg"() -> (w229:dbl)
              n97 = for {
                tunnel: w210 -> [w281]
                tunnel: w241 -> [w280] mode=indexing
                shift-right: [w277] -> _
                shift-left: 0 -> [w279]
                tunnel: [w277] -> w238 mode=indexing
                n98 = Threshold 1D Array(1:w279, 2:w280, 3:w281) -> (0:w278:dbl)
                n99 = To Long Integer(number=w278) -> (32bit integer=w277:i32)
              }
              n100 = Index Array(array=w238) -> (element=w237:i32)  [unwired: 1 in]
              n101 = Array Subset(array=w238, index=1) -> (w236:i32[])  [unwired: 1 in]
              n102 = for {
                shift-right: [w275] -> _
                shift-left: w237 -> [w276]
                tunnel: w236 -> [w275] mode=indexing
                tunnel: w235 -> [w273]
                tunnel: w231 -> [w271]
                tunnel: [w267] -> w226 mode=indexing
                tunnel: [w270] -> w223 mode=indexing
                tunnel: w230 -> [w269]
                tunnel: w229 -> [w268]
                tunnel: [w266] -> w220 mode=concatenating
                tunnel: [w265] -> w217 mode=concatenating
                tunnel: [w264] -> w216 mode=concatenating
                n103 = Subtract(x=w275, y=w276) -> (x-y=w274:i32)
                n104 = Array Subset(array=w273, index=w276, length=w274) -> (w272:dbl[])
                n105 = call "WT_Single_Pass_analysis.vi"("Displacement"=w272, "Start Cut Deg"=w269, "End Cut Deg"=w268, "Radius"=w271) -> ("Blade Angles"=w267:dbl[], "Blade Positions"=w270:dbl[], "Blade1"=w266:dbl[], "Blade 2"=w265:dbl[], "Blade 3"=w264:dbl[])  [unwired: 1 in]
              }
              n106 = case shown="1" w227 {
                tunnel: w226 -> [w258 w263]
                tunnel: w225 -> [w257 _]
                tunnel: [w256 w263] -> w224
                tunnel: w223 -> [w255 w262]
                tunnel: w222 -> [w254 _]
                tunnel: [w253 w262] -> w221
                tunnel: w220 -> [w252 w261]
                tunnel: [w250 w261] -> w219
                tunnel: w218 -> [w251 _]
                tunnel: w217 -> [w249 w260]
                tunnel: w216 -> [w248 w259]
                tunnel: w215 -> [w247 _]
                tunnel: [w246 w260] -> w214
                tunnel: w213 -> [w245 _]
                tunnel: [w244 w259] -> w212
                frame 2, Default {
                  n107 = Build Array (concatenate)(w258, w257) -> (w256:dbl[][])
                  n108 = Build Array (concatenate)(w251, w252) -> (w250:dbl[])
                  n109 = Build Array (concatenate)(w247, w249) -> (w246:dbl[])
                  n110 = Build Array (concatenate)(w245, w248) -> (w244:dbl[])
                  n111 = Build Array (concatenate)(w255, w254) -> (w253:dbl[][])
                }
                frame 1 {
                }
              }
            }
            "Blade 1 Every Pass" <- w203
            "Blade 3 Every Pass" <- w201
            "Blade 2 Every Pass" <- w202
          }
          frame #1 {
            n112 = Transpose 2D Array(2D array=w286) -> (transposed array=w283:dbl[][])
            "Blade Angles" <- w283
            n113 = Transpose 2D Array(2D array=w285) -> (transposed array=w284:dbl[][])
            "Blade Positions" <- w284
            n114 = for {
              tunnel: w283 -> [w294] mode=indexing
              tunnel: w284 -> [w293] mode=indexing
              tunnel: [w287] -> w282 mode=indexing
              n115 = call <vilib>:"Std Deviation and Variance.vi"("X"=w294) -> ("mean"=w292:dbl, "variance"=w291:dbl)  [unwired: 1 in, 1 out]
              n116 = call <vilib>:"Std Deviation and Variance.vi"("X"=w293) -> ("mean"=w290:dbl, "variance"=w289:dbl)  [unwired: 1 in, 1 out]
              n117 = Build Array(w292, w291, w290, w289) -> (w288:dbl[])
              n118 = Number To Fractional String(number=w288) -> (F-format string=w287:string[])  [unwired: 3 in]
            }
            "Blade Analysis" <- w282
          }
        }
      }
      frame "Phase locked Stats" {
        # "N"
        # "U2T"
        # "UT"
        # "T"
        n119 = while {
          tunnel: w306 -> [w310]
          tunnel: w305 -> [w312]
          tunnel: w300 -> [w327]
          shift-right: [w316] -> _
          shift-left: _ -> [w322]
          tunnel: w301 -> [w309]
          shift-right: [w315] -> _
          shift-left: _ -> [w321]
          shift-right: [w314] -> _
          shift-left: _ -> [w320]
          shift-right: [w313] -> _
          shift-left: _ -> [w319]
          tunnel: w299 -> [w328]
          tunnel: [w318] -> w298
          tunnel: [w317] -> w296
          stop <- TRUE stop-if-true
          n120 = case shown="2, Default" w328 {
            tunnel: w310 -> [_ w340]
            tunnel: w327 -> [_ w339]
            tunnel: [w336 w337] -> w326
            tunnel: [w335 w337] -> w325
            tunnel: [w334 w337] -> w324
            tunnel: [w333 w337] -> w323
            tunnel: w322 -> [w336 _]
            tunnel: w321 -> [w335 _]
            tunnel: w320 -> [w334 _]
            tunnel: w319 -> [w333 _]
            frame 2, Default {
            }
            frame 1 {
              n121 = Array Size(array=w339) -> (size(s)=w338:i32)
              n122 = Initialize Array(0.0, w338, w340) -> (w337:dbl[][])
            }
          }
          n123 = Array Size(array=w309) -> (size(s)=w308:i32)
          n124 = for {
            N: w310 -> [_]
            tunnel: w312 -> [w331]
            tunnel: [w330] -> w311 mode=indexing
            i -> [w332]
            n125 = Multiply(x=w332, y=w331) -> (x*y=w330:dbl)
          }
          "X array" <- w311
          n126 = property on="Channel to Phase lock" class="LstBox (strict)"() -> ("Item Names"=w307:string[])  [unwired: 2 in, 2 out]
          n127 = for {
            tunnel: w310 -> [w370]
            tunnel: w312 -> [_]
            tunnel: w327 -> [w343] mode=indexing
            tunnel: w309 -> [w367]
            tunnel: w326 -> [w356] mode=indexing
            tunnel: [w352] -> w316 mode=indexing
            tunnel: [w351] -> w315 mode=indexing
            tunnel: [w350] -> w314 mode=indexing
            tunnel: [w349] -> w313 mode=indexing
            tunnel: w325 -> [w355] mode=indexing
            tunnel: w324 -> [w354] mode=indexing
            tunnel: w323 -> [w353] mode=indexing
            tunnel: [w359] -> w318 mode=indexing
            tunnel: [w357] -> w317 mode=indexing
            tunnel: w311 -> [w348]
            tunnel: w308 -> [_]
            tunnel: w307 -> [w346]
            i -> [w347]
            # "u^2"
            # "U"
            # "U2T"
            # "UT"
            # "T"
            n128 = To Long Integer(number=w370) -> (32bit integer=w369:i32)
            n129 = Index Array(array=w346, index=w343) -> (element=w345:string)
            n130 = property on="Inst Channels" class="XYGraph (strict)"("Active Plot"=w347, "Plot.Plot Name"=w345) -> ()  [unwired: 2 in, 2 out]
            n131 = local read "WT Revolution Start times"() -> (w374:dbl[])
            n132 = Index Array(array=w367, index=w343) -> (element=w344:T6)
            n133 = Unbundle By Name(w344) -> ("Eng Values"=w368:dbl[], "Weighting"=w366:dbl[])
            n134 = call "Get Time Trace.vi"("Channel Index"=w343) -> ("Time (s)"=w342:dbl[])  [unwired: 1 out]
            n135 = call "Create_Bin_Indices.vi"("No Of Bins"=w369, "Cycle Start TIme"=w374) -> ("Bin Number"=w372:i32[], "Bin Start Time"=w373:dbl[])
            n136 = for {
              tunnel: w373 -> [w406]
              tunnel: w342 -> [w405] mode=indexing
              shift-right: [w402] -> _
              shift-left: 0 -> [w399]
              tunnel: w372 -> [w403]
              tunnel: [w401] -> w371 mode=indexing
              n137 = Threshold 1D Array(1:w399, 2:w405, 3:w406) -> (0:w404:dbl)
              n138 = Round Toward -Infinity(1:w404) -> (0:w400:dbl)
              n139 = To Long Integer(number=w400) -> (32bit integer=w402:i32)
              n140 = Index Array(array=w403, index=w402) -> (element=w401:i32)
            }
            n141 = for {
              tunnel: w371 -> [w385] mode=indexing
              tunnel: w368 -> [w377] mode=indexing
              tunnel: w366 -> [w376] mode=indexing
              shift-right: [w381] -> w352
              shift-left: w356 -> [w386]
              shift-right: [w380] -> w351
              shift-left: w355 -> [w382]
              shift-right: [w379] -> w350
              shift-left: w354 -> [w383]
              shift-right: [w378] -> w349
              shift-left: w353 -> [w384]
              n142 = in-place {
                in-place-border: w377 -> [w391]
                in-place-border: w376 -> [w394]
                n143 = in-place-array #1(w383, w385) -> (w388:dbl)
                n144 = in-place-array #2(w386, w385) -> (w398:dbl)
                n145 = in-place-array #3(w382, w385) -> (w396:dbl)
                n146 = in-place-array #4(w384, w385) -> (w387:dbl)
                n147 = Add(x=w394, y=w396) -> (x+y=w395:dbl)
                n148 = Multiply(x=w391, y=w394) -> (x*y=w393:dbl)
                n149 = Add(x=w393, y=w388) -> (x+y=w389:dbl)
                n150 = Multiply(x=w391, y=w393) -> (x*y=w392:dbl)
                n151 = Increment(x=w398) -> (x+1=w397:dbl)
                n152 = Add(x=w392, y=w387) -> (x+y=w390:dbl)
                n153 = in-place-array #1(w389) -> (w379:dbl[])  [unwired: 1 out]
                n154 = in-place-array #2(w397) -> (w381:dbl[])  [unwired: 1 out]
                n155 = in-place-array #3(w395) -> (w380:dbl[])  [unwired: 1 out]
                n156 = in-place-array #4(w390) -> (w378:dbl[])  [unwired: 1 out]
              }
            }
            n157 = Divide(x=w349, y=w352) -> (x/y=w363:dbl[])
            n158 = Divide(x=w350, y=w352) -> (x/y=w365:dbl[])
            n159 = Divide(x=w351, y=w352) -> (x/y=w364:dbl[])
            n160 = Divide(x=w363, y=w364) -> (x/y=w362:dbl[])
            n161 = Divide(x=w365, y=w364) -> (x/y=w358:dbl[])
            n162 = Square(x=w358) -> (x^2=w361:dbl[])
            n163 = Subtract(x=w362, y=w361) -> (x-y=w360:dbl[])
            n164 = Bundle(w358, w360) -> (w359:cluster{dbl[], dbl[]})  [unwired: 1 in]
            n165 = Bundle(w348, w358) -> (w357:cluster{dbl[], dbl[]})  [unwired: 1 in]
          }
        }
        "Inst Channels" <- w296
      }
      frame "Cross correlation phase locking" {
        n166 = disable-structure shown="Disabled" {
          disable-tunnel: w412 -> [w424 _]
          disable-tunnel: w411 -> [w423 _]
          disable-tunnel: w410 -> [w422 _]
          disable-tunnel: w409 -> [w421 _]
          disable-tunnel: w408 -> [w419 _]
          frame Disabled {
            n167 = To Long Integer(number=w421) -> (32bit integer=w420:i32)
            n168 = stacked-sequence {
              seq-local: [w426 _] -> [_ w484]
              seq-local: [w425 _] -> [_ w483]
              tunnel: w424 -> [w430 _]
              tunnel: w423 -> [w429 _]
              tunnel: w422 -> [w428 _]
              tunnel: w420 -> [w427 w482]
              tunnel: w419 -> [_ w479]
              frame #0 {
                n169 = while {
                  shift-right: [w445] -> _
                  shift-left: _ -> [w444]
                  tunnel: w430 -> [w441]
                  tunnel: w429 -> [w440]
                  tunnel: w428 -> [w439]
                  tunnel: w427 -> [w436]
                  tunnel: [w434] -> w426
                  tunnel: [w433] -> w425
                  shift-right: [w431] -> _
                  shift-left: _ -> [w432]
                  stop <- TRUE stop-if-true
                  n170 = local read "WT Revolution Start times"() -> (w437:dbl[])
                  n171 = local read "X array"() -> (w443:dbl[])
                  n172 = for {
                    tunnel: [w475] -> w445 mode=indexing
                    tunnel: w444 -> [w474]
                    tunnel: w443 -> [w472]
                    tunnel: [w470] -> w434 mode=indexing
                    tunnel: "Cross_Corr to Phase Lock" -> [w469] mode=indexing
                    tunnel: w441 -> [w468]
                    tunnel: w440 -> [w466]
                    tunnel: w439 -> [w464]
                    tunnel: w437 -> [w461]
                    tunnel: w436 -> [w460]
                    tunnel: "Time Shift" -> [w457]
                    tunnel: [w451] -> w433 mode=indexing
                    tunnel: w432 -> [w449]
                    tunnel: [w448] -> w431 mode=indexing
                    i -> [w447]
                    w450 = 0 items=["nearest", "linear", "spline", "cubic Hermite", "Lagrange"] ("interp. method")
                    n173 = Index Array(array=w468, index (row)=w469) -> (element=w467:i32[])  [unwired: 1 in]
                    n174 = Index Array(array=w474, index (row)=w447) -> (element=w473:T8[])  [unwired: 1 in]
                    n175 = Index Array(array=w449, index (row)=w447) -> (element=w446:T9[])  [unwired: 1 in]
                    n176 = Index Array(array=w467) -> (element #1=w463:i32, element #2=w462:i32)  [unwired: 2 in]
                    n177 = Index Array(array=w466, index=w463) -> (element=w459:T6)
                    n178 = Index Array(array=w464, index=w463) -> (element=w456:T3)
                    n179 = Index Array(array=w466, index=w462) -> (element=w465:T6)
                    n180 = Index Array(array=w464, index=w462) -> (element=w455:T3)
                    n181 = in-place {
                      in-place-border: w457 -> [w478]
                      n182 = in-place-cluster #5(w459) -> ("Time (s)"=w477:dbl[])
                      n183 = Add(x=w478, y=w477) -> (x+y=w476:dbl[])
                      n184 = in-place-cluster #5("Time (s)"=w476) -> (w458:T6)
                    }
                    n185 = Unbundle By Name(w456) -> ("Inst name"=w454:string)
                    n186 = Unbundle By Name(w455) -> ("Inst name"=w453:string)
                    n187 = call "Phase_Av_Weighted_Cross_Moments.vi"("AI Cluster 1"=w456, "WT Revolution Start times"=w461, "interp. method"=w450, "Time Cluster 1"=w458, "AI Cluster 2"=w455, "Time Cluster 2"=w465, "Shift In"=w473, "Shift Cluster In"=w446, "No Of Bins"=w460) -> ("Phase locked uw/u'w'"=w471:dbl[], "Shift Cluster Out"=w448:T9[], "Shift Out"=w475:T8[])  [unwired: 3 in, 1 out]
                    n188 = Format Into String(format string="%s & %s", w454, w453) -> (resulting string=w451:string)  [unwired: 2 in, 1 out]
                    n189 = Bundle("X array"=w472, "Phase locked uw/u'w'"=w471) -> (w470:T10)  [unwired: 1 in]
                  }
                  "Cross Chs" <- w434
                }
              }
              frame #1 {
                n190 = local read "Add Phase data to results file"() -> (w480:bool)
                n191 = Compound Arithmetic op=AND(w480, w479) -> (w481:bool)
                n192 = case shown="True" w481 {
                  tunnel: w484 -> [_ w487]
                  tunnel: w483 -> [_ w486]
                  tunnel: w482 -> [_ w485]
                  frame False {
                  }
                  frame True {
                    n193 = stacked-sequence {
                      tunnel: w485 -> [w490 _]
                      tunnel: w487 -> [_ w507]
                      tunnel: w486 -> [w488 _]
                      frame #0 {
                        n194 = local read "Plug in titles"() -> (w491:string[])
                        n195 = Divide(x=360, y=w490) -> (x/y=w493:dbl)
                        n196 = Increment(x=w490) -> (x+1=w489:i32)
                        n197 = for {
                          tunnel: w488 -> [w500] mode=indexing
                          tunnel: w493 -> [w499]
                          shift-right: [w496] -> w492
                          shift-left: w491 -> [w498]
                          tunnel: w489 -> [w495]
                          n198 = for {
                            N: w495 -> [_]
                            tunnel: w500 -> [w502]
                            tunnel: w499 -> [w505]
                            tunnel: [w503] -> w497 mode=indexing
                            i -> [w506]
                            n199 = Multiply(x=w505, y=w506) -> (x*y=w501:dbl)
                            n200 = Format Into String(format string="%s:Mean:%.1f Deg:%.1f", w502, w501, w501) -> (resulting string=w503:string)  [unwired: 2 in, 1 out]
                          }
                          n201 = Build Array (concatenate)(w498, w497) -> (w496:string[])
                        }
                        n202 = local write "Plug in titles"(w492) -> ()
                      }
                      frame #1 {
                        n203 = local read "Plug in values"() -> (w509:string[])
                        n204 = for {
                          tunnel: w507 -> [w511] mode=indexing
                          shift-right: [w513] -> w508
                          shift-left: w509 -> [w514]
                          n205 = Unbundle(w511) -> ("Phase locked uw/u'w'"=w510:dbl[])  [unwired: 1 out]
                          n206 = for {
                            tunnel: w510 -> [w515] mode=indexing
                            tunnel: [w516] -> w512 mode=indexing
                            n207 = call "Number_2_string.vi"("number"=w515) -> ("String"=w516:string)  [unwired: 1 in]
                          }
                          n208 = Build Array (concatenate)(w514, w512) -> (w513:string[])
                        }
                        n209 = local write "Plug in values"(w508) -> ()
                      }
                    }
                  }
                }
              }
            }
          }
          frame Enabled {
          }
        }
      }
      frame "Output WT Statistics" {
        n210 = property on="Turbine to Phase Lock to" class="Ring (strict)"() -> ("Strings []"=w534:string[])  [unwired: 2 in, 2 out]
        n211 = for {
          shift-right: [w561] -> w526
          shift-left: "WT" -> [w562]
          tunnel: w534 -> [w552] mode=indexing
          tunnel: [w557] -> w533 mode=indexing
          n212 = String Subset(string=w552, offset (0)=6, length (rest)=1 ("length (rest)")) -> (substring=w548:string)
          n213 = String Subset(string=w552, offset (0)=7, length (rest)=1 ("length (rest)")) -> (substring=w547:string)
          n214 = Equal?(x=")", y=w547) -> (x = y?=w550:bool)
          n215 = case shown="True" w550 {
            tunnel: [w564 w567] -> w549
            tunnel: w548 -> [w566 w567]
            tunnel: w547 -> [w565 _]
            frame False {
              n216 = Concatenate Strings(w566, w565) -> (w564:string)
            }
            frame True {
            }
          }
          n217 = Equal?(x=")", y=w548) -> (x = y?=w558:bool)
          n218 = Select(t="1", s=w558, f=w549) -> (s? t:f=w557:string)
          n219 = Concatenate Strings(w562, "_", w557) -> (w561:string)
        }
        "WT Numbers" <- w533
        n220 = local read "All WTs"() -> (w532:dbl[][])
        n221 = Build Array(w526) -> (w524:string[])
        n222 = Build Array("Wind:Turbines:Logged") -> (w525:string[])
        n223 = for {
          tunnel: w532 -> [w579] mode=indexing
          shift-right: [w573] -> w522
          shift-left: w524 -> [w574]
          shift-right: [w568] -> w523
          shift-left: w525 -> [w571]
          tunnel: string[] ["WT_%s:Hub_RPM:Mean", "WT_%s:Hub_RPM:St_Dev", "WT_%s:Hub_RPM:Max-Min", "WT_%s:Number_of:Revs"] ("Plug in titles") -> [w572]
          tunnel: w533 -> [w569] mode=indexing
          n224 = Index Array(array=w579, index=0) -> (element=w578:dbl)
          n225 = Index Array(array=w579, index=1) -> (element=w577:dbl)
          n226 = Index Array(array=w579, index=2) -> (element=w576:dbl)
          n227 = Index Array(array=w579, index=3) -> (element=w575:dbl)
          n228 = for {
            tunnel: w572 -> [w590] mode=indexing
            tunnel: [w589] -> w570 mode=indexing
            tunnel: w569 -> [w588]
            n229 = Format Into String(format string=w590, w588) -> (resulting string=w589:string)  [unwired: 2 in, 1 out]
          }
          n230 = call "Number_2_string.vi"("number"=w578) -> ("String"=w586:string)  [unwired: 1 in]
          n231 = call "Number_2_string.vi"("number"=w577) -> ("String"=w587:string)  [unwired: 1 in]
          n232 = call "Number_2_string.vi"("number"=w576) -> ("String"=w585:string)  [unwired: 1 in]
          n233 = Number To Decimal String(number=w575) -> (decimal integer string=w584:string)  [unwired: 1 out]
          n234 = Build Array (concatenate)(w574, w586, w587, w585, w584) -> (w573:string[])
          n235 = Build Array (concatenate)(w571, w570) -> (w568:string[])
        }
        n236 = Decimal String To Number(string=w533) -> (number=w530:i32[])  [unwired: 2 in, 1 out]
        n237 = Index Array(array=w532, index (col)=0 ("disabled index (col)")) -> (element=w529:dbl[])  [unwired: 1 in]
        n238 = local read "Laser Disp Index"() -> (w544:i32)
        n239 = Bundle(w530, "All WTs"=w529) -> (→"Turbine RPMs":cluster{i32[], "All WTs":dbl[]})  [unwired: 1 in]
        n240 = Greater Or Equal To 0?(x=w544) -> (x >= 0?=w543:bool)
        n241 = local read "Plug in values"() -> (w520:string[])
        n242 = local read "Plug in titles"() -> (w521:string[])
        n243 = Build Array (concatenate)(w523, w521) -> (→"Plug in titles":string[])
        n244 = Build Array (concatenate)(w522, w520) -> (→"Plug in values":string[])
        n245 = Select(t="Laser Displacement Analysis", s=w543, f="Get Last Block info") -> (s? t:f=w542:string)
      }
      frame "Laser Displacement Analysis" {
        # "L"
        # "S"
        # "R"
        # "D^2"
        # "D"
        n246 = stacked-sequence {
          seq-local: [_ w609 _ _ _ _ _] -> [_ _ w627 _ _ _ _]
          seq-local: [_ _ w628 _ _ _ _] -> [_ _ _ _ w694 _ _]
          seq-local: [w602 _ _ _ _ _ _] -> [_ _ _ _ w690 _ _]
          seq-local: [w603 _ _ _ _ _ _] -> [_ _ _ _ w689 _ _]
          seq-local: [_ _ _ w664 _ _ _] -> [_ _ _ _ w682 _ _]
          seq-local: [_ _ _ w659 _ _ _] -> [_ _ _ _ w681 _ _]
          seq-local: [_ _ _ w662 _ _ _] -> [_ _ _ _ w680 _ _]
          seq-local: [w603 _ _ _ _ _ _] -> [_ w610 _ _ _ _ _]
          tunnel: w601 -> [_ _ _ _ _ _ _]
          tunnel: w600 -> [_ _ _ w660 w683 _ _]
          tunnel: w599 -> [_ _ _ _ _ w768 w806]
          tunnel: [_ _ _ _ _ TRUE _] -> w598
          tunnel: [_ _ _ _ _ "Get Last Block info" _] -> w597
          tunnel: w593 -> [w606 w613 _ _ _ _ _]
          tunnel: w592 -> [_ _ _ w678 _ _ _]
          frame #0 {
            n247 = local read "Laser Phase lock index"() -> (w604:i32)
            n248 = Index Array(array=w606, index=w604) -> (element=w605:cluster{dbl[], dbl[]})
            n249 = Unbundle(w605) -> (w603:dbl[], w602:dbl[])
            n250 = Build Array (concatenate)(w603, w603, 0.0) -> ()  [unwired: 1 out]
            n251 = Build Array (concatenate)(w602, w602, 0.0) -> ()  [unwired: 1 out]
          }
          frame #1 {
            n252 = local read "Laser Status Index"() -> (w612:i32)
            n253 = Less Than 0?(x=w612) -> (x < 0?=w611:bool)
            n254 = case shown="True" w611 {
              tunnel: w613 -> [w619 _]
              tunnel: w610 -> [_ w626]
              tunnel: [w615 w621] -> w609
              frame False {
                n255 = local read "L Status Phase lock index"() -> (w618:i32)
                n256 = Index Array(array=w619, index=w618) -> (element=w620:cluster{dbl[], dbl[]})
                n257 = Unbundle(w620) -> (w614:dbl[])  [unwired: 1 out]
                n258 = Build Array (concatenate)(w614, w614, 0.0) -> ()  [unwired: 1 out]
                n259 = Greater?(x=w614, y=0.4) -> (0:w615:bool[])
              }
              frame True {
                n260 = Greater?(x=w626, y=-5) -> (0:w622:bool[])
                n261 = Build Array (concatenate)(w622, w622, FALSE) -> (w623:bool[])
                n262 = Not(x=w623) -> (.not. x?=w621:bool[])
              }
            }
          }
          frame #2 {
            n263 = Index Array(array=w627, index=0) -> (element=w630:bool)
            n264 = for {
              tunnel: w627 -> [w637] mode=indexing
              shift-right: [w637] -> _
              shift-left: w630 -> [w632]
              shift-right: [w634] -> w628
              shift-left: i32[] [] -> [w635]
              i -> [w636]
              n265 = Not Equal?(x=w637, y=w632) -> (x != y?=w633:bool)
              n266 = case shown="True" w633 {
                tunnel: w636 -> [_ w644]
                tunnel: w635 -> [w638 w642]
                tunnel: [w638 w643] -> w634
                tunnel: w632 -> [_ w639]
                frame False {
                }
                frame True {
                  n267 = Array Size(array=w642) -> (size(s)=w641:i32)
                  n268 = Equal To 0?(x=w641) -> (x = 0?=w640:bool)
                  n269 = case shown="True" w640 {
                    tunnel: w644 -> [w645 w651]
                    tunnel: w642 -> [w647 w650]
                    tunnel: [w646 w649] -> w643
                    tunnel: w639 -> [_ w648]
                    frame False {
                      n270 = Build Array (concatenate)(w647, w645) -> (w646:i32[])
                    }
                    frame True {
                      n271 = case shown="False" w648 {
                        tunnel: w651 -> [_ w655]
                        tunnel: w650 -> [w652 w654]
                        tunnel: [w652 w653] -> w649
                        frame False {
                        }
                        frame True {
                          n272 = Build Array (concatenate)(w654, w655) -> (w653:i32[])
                        }
                      }
                    }
                  }
                }
              }
            }
          }
          frame #3 {
            n273 = local read "Laser Disp Index"() -> (w677:i32)
            n274 = Index Array(array=w678, index=w677) -> (element=w679:T3)
            n275 = Unbundle By Name(w679) -> ("Y"=w670:dbl)
            n276 = Absolute Value(x=w670) -> (abs(x)=w664:dbl)
            n277 = formula code="S=(0.0001*R*R) -0.0619*R+7.7094;"("R"=w664) -> ("S"=w658:dbl)
            n278 = Divide(x=10, y=w664) -> (x/y=w675:dbl)
            n279 = Inverse Tangent(1:w675) -> (0:w674:dbl)
            n280 = Divide(x=w674, y=3.141592653589793) -> (x/y=w672:dbl)
            n281 = Max & Min(x=w658, y=0.0) -> (max(x,y)=w656:dbl)  [unwired: 1 out]
            n282 = Divide(x=w656, y=w664) -> (x/y=w665:dbl)
            n283 = Inverse Tangent(1:w665) -> (0:w666:dbl)
            n284 = Divide(x=w666, y=3.141592653589793) -> (x/y=w668:dbl)
            n285 = Multiply(x=w672, y=180.0) -> (x*y=w661:dbl)
            n286 = Multiply(x=w668, y=180.0) -> (x*y=w663:dbl)
            n287 = Divide(x=w663, y=w660) -> (x/y=w662:dbl)
            n288 = Divide(x=w661, y=w660) -> (x/y=w659:dbl)
          }
          frame #4 {
            w684 = 360.0 ("y")
            n289 = Divide(x="Start Cut Deg", y=w683) -> (x/y=w696:dbl)
            n290 = Divide(x="End Cut Deg", y=w683) -> (x/y=w697:dbl)
            n291 = To Long Integer(number=w696) -> (32bit integer=w692:i32)
            n292 = To Long Integer(number=w697) -> (32bit integer=w695:i32)
            n293 = Add(x=w692, y=w695) -> (x+y=w691:i32)
            n294 = Divide(x=w683, y=w684) -> (x/y=w688:dbl)
            n295 = Multiply(x=w688, y=6.283185307179586) -> (x*y=w687:dbl)
            n296 = Multiply(x=w687, y=w682) -> (x*y=w685:dbl)
            n297 = for {
              N: 3 -> [_]
              tunnel: w689 -> [w735]
              tunnel: w694 -> [w732]
              tunnel: w692 -> [w702]
              tunnel: w691 -> [w728]
              tunnel: w685 -> [w727]
              tunnel: w690 -> [w719]
              tunnel: w684 -> [w712]
              tunnel: w683 -> [w706]
              tunnel: w681 -> [w704]
              tunnel: w680 -> [w700]
              i -> [w726]
              n298 = Multiply(x=w726, y=2) -> (x*y=w730:i32)
              n299 = Increment(x=w730) -> (x+1=w729:i32)
              n300 = Index Array(array=w732, index=w730) -> (element=w737:i32)
              n301 = Index Array(array=w732, index=w729) -> (element=w738:i32)
              n302 = Subtract(x=w738, y=w737) -> (x-y=w736:i32)
              n303 = Add(x=w700, y=w702) -> (x+y=w701:dbl)
              n304 = Add(x=w737, y=w701) -> (x+y=w722:dbl)
              n305 = Subtract(x=w736, y=w728) -> (x-y=w705:i32)
              n306 = Max & Min(x=w705, y=w704) -> (min(x,y)=w703:dbl)  [unwired: 1 out]
              n307 = Array Subset(array=w719, index=w722, length=w703) -> (w710:dbl[])
              n308 = call-poly <vilib>:"Mean.vi"("X"=w710) -> ("mean"=w709:dbl)  [unwired: 1 out]
              n309 = Multiply(x=2.0, y=w709) -> (x*y=w707:dbl)
              n310 = call "Top_and_Tail_ph.vi"("Array in"=w710, "Threshold"=w707) -> ("Length"=w717:i32, "Start Index"=w721:i32)
              n311 = Add(x=w722, y=w721) -> (x+y=w718:dbl)
              n312 = Array Subset(array=w719, index=w718, length=w717) -> (w720:dbl[])
              n313 = call-poly <vilib>:"Mean.vi"("X"=w720) -> ("mean"=w723:dbl)  [unwired: 1 out]
              n314 = Array Subset(array=w735, index=w718, length=w717) -> (w725:dbl[])
              n315 = Array Size(array=w725) -> (size(s)=w734:i32)
              n316 = for {
                N: w734 -> [_]
                tunnel: w727 -> [w765]
                tunnel: [w763] -> w733 mode=indexing
                i -> [w764]
                n317 = Multiply(x=w764, y=w765) -> (x*y=w763:dbl)
              }
              n318 = call <vilib>:"Linear Fit.vi"("Y"=w725, "X"=w733) -> ("slope"=w716:dbl)  [unwired: 9 in, 4 out]
              n319 = call-poly <vilib>:"Mean.vi"("X"=w725) -> ("mean"=w724:dbl)  [unwired: 1 out]
              n320 = Inverse Tangent(1:w716) -> (0:w715:dbl)
              n321 = Divide(x=w715, y=6.283185307179586) -> (x/y=w713:dbl)
              n322 = Multiply(x=w713, y=w712) -> (x*y=w711:dbl)
              n323 = case shown="0, Default" w726 {
                tunnel: w725 -> [w742 w749 w756]
                tunnel: w716 -> [w746 w753 w761]
                tunnel: w724 -> [w745 w754 w762]
                tunnel: w720 -> [_ _ _]
                tunnel: w723 -> [w744 w752 w760]
                tunnel: w711 -> [w743 w751 w759]
                tunnel: w706 -> [w739 w750 w757]
                frame 0, Default {
                  n324 = Bundle(0.0, "Angular Step(deg)"=w739, w742) -> (→"Mean Blade 1":cluster{dbl, "Angular Step(deg)":dbl, dbl[]})  [unwired: 1 in]
                  "slope 1" <- w746
                  "Av Disp 1" <- w745
                  "Av Variance 1" <- w744
                  "Angle 1" <- w743
                }
                frame 1 {
                  n325 = Bundle(0.0, "Angular Step(deg)"=w750, w749) -> (→"Mean Blade 2":cluster{dbl, "Angular Step(deg)":dbl, dbl[]})  [unwired: 1 in]
                  "Av Disp 2" <- w754
                  "slope 2" <- w753
                  "Av Variance 2" <- w752
                  "Angle 2" <- w751
                }
                frame 2 {
                  n326 = Bundle(0.0, "Angular Step(deg)"=w757, w756) -> (→"Mean Blade 3":cluster{dbl, "Angular Step(deg)":dbl, dbl[]})  [unwired: 1 in]
                  "Av Disp 3" <- w762
                  "slope 3" <- w761
                  "Av Variance 3" <- w760
                  "Angle 3" <- w759
                }
              }
            }
          }
          frame #5 {
            n327 = case shown="True" w768 {
              frame False {
              }
              frame True {
                n328 = for {
                  N: 3 -> [_]
                  tunnel: [w799] -> w790 mode=indexing
                  tunnel: [w798] -> w789 mode=indexing
                  tunnel: [w797] -> w788 mode=indexing
                  tunnel: [w796] -> w772 mode=indexing
                  i -> [w805]
                  n329 = Increment(x=w805) -> (x+1=w804:i32)
                  n330 = Format Into String(format string="Blade %d:", w804) -> (resulting string=w795:string)  [unwired: 2 in, 1 out]
                  n331 = Concatenate Strings(w795, "Angle:") -> (w796:string)
                  n332 = Concatenate Strings(w795, "Slope:") -> (w799:string)
                  n333 = Concatenate Strings(w795, "Average:X") -> (w798:string)
                  n334 = Concatenate Strings(w795, "Variance of:X") -> (w797:string)
                }
                n335 = local read "Av Variance 1"() -> (w779:dbl)
                n336 = local read "Av Variance 2"() -> (w778:dbl)
                n337 = local read "Av Variance 3"() -> (w777:dbl)
                n338 = local read "Av Disp 1"() -> (w782:dbl)
                n339 = local read "Av Disp 2"() -> (w781:dbl)
                n340 = local read "Av Disp 3"() -> (w780:dbl)
                n341 = local read "Angle 3"() -> (w771:dbl)
                n342 = local read "slope 1"() -> (w785:dbl)
                n343 = local read "slope 2"() -> (w784:dbl)
                n344 = local read "slope 3"() -> (w783:dbl)
                n345 = local read "Angle 1"() -> (w770:dbl)
                n346 = local read "Angle 2"() -> (w769:dbl)
                n347 = Build Array(w770, w769, w771, w785, w784, w783, w782, w781, w780, w779, w778, w777) -> (w776:dbl[])
                n348 = local read "Plug in values"() -> (w775:string[])
                n349 = local read "Plug in titles"() -> (w787:string[])
                n350 = for {
                  tunnel: w776 -> [w793] mode=indexing
                  tunnel: [w792] -> w774 mode=indexing
                  n351 = call "Number_2_string.vi"("number"=w793) -> ("String"=w792:string)  [unwired: 1 in]
                }
                n352 = Build Array (concatenate)(w787, w772, w790, w789, w788) -> (w786:string[])
                n353 = Build Array (concatenate)(w775, w774) -> (w773:string[])
                n354 = local write "Plug in titles"(w786) -> ()
                n355 = local write "Plug in values"(w773) -> ()
              }
            }
          }
          frame #6 {
            n356 = case shown="True" w806 {
              frame False {
              }
              frame True {
                n357 = local read "Blade Analysis"() -> (w810:string[][])
                n358 = for {
                  tunnel: [w815] -> w813 mode=concatenating
                  tunnel: w810 -> [w814] mode=indexing
                  tunnel: [w814] -> w807 mode=concatenating
                  i -> [w827]
                  n359 = Increment(x=w827) -> (x+1=w826:i32)
                  n360 = Format Into String(format string="Blade %d:", w826) -> (resulting string=w821:string)  [unwired: 2 in, 1 out]
                  n361 = Concatenate Strings(w821, "Angle:Degrees") -> (w819:string)
                  n362 = Concatenate Strings(w821, "Angle:Variance") -> (w818:string)
                  n363 = Concatenate Strings(w821, "Position:(mm)") -> (w817:string)
                  n364 = Concatenate Strings(w821, "Position:Variance") -> (w816:string)
                  n365 = Build Array(w819, w818, w817, w816) -> (w815:string[])
                }
                n366 = local read "Plug in titles"() -> (w812:string[])
                n367 = local read "Plug in values"() -> (w809:string[])
                n368 = Build Array (concatenate)(w812, w813) -> (w811:string[])
                n369 = Build Array (concatenate)(w809, w807) -> (w808:string[])
                n370 = local write "Plug in values"(w808) -> ()
                n371 = local write "Plug in titles"(w811) -> ()
              }
            }
          }
        }
      }
      frame "Get Last Block info" {
        n372 = case shown="\"Take New Data\"" w838 {
          tunnel: [w848 "Post Process"] -> w837
          tunnel: [w851 TRUE ("Processing last block?")] -> w836
          tunnel: w835 -> [w851 _]
          tunnel: w830 -> [w847 _]
          tunnel: w829 -> [w846 _]
          frame "Take New Data" {
            n373 = local read "WT Numbers"() -> (w845:string[])
            n374 = for {
              tunnel: w847 -> [w861]
              tunnel: w846 -> [w860]
              tunnel: w845 -> [w859] mode=indexing
              tunnel: [w856] -> w842 mode=concatenating
              n375 = Format Into String(format string=w861, w859) -> (resulting string=w858:string)  [unwired: 2 in, 1 out]
              n376 = Format Into String(format string=w860, w859) -> (resulting string=w857:string)  [unwired: 2 in, 1 out]
              n377 = Build Array(w858, w857) -> (w856:string[])
            }
            n378 = call "Get_ADAM_Ch_names_client.vi"("Channel names set"=Channel_names."Active Only") -> ("Ch names"=w843:string[])
            n379 = for {
              tunnel: w843 -> [w855]
              tunnel: w842 -> [w854] mode=indexing
              tunnel: [w852] -> w840
              stop <- w852 continue-if-true
              n380 = Search 1D Array(1D array=w855, element=w854) -> (index of element=w853:i32)  [unwired: 1 out]
              n381 = Greater Or Equal To 0?(x=w853) -> (x >= 0?=w852:bool)
            }
            n382 = And(x=w840, y="Change Dem Voltages?") -> (x .and. y?=w839:bool)
            n383 = Select(t="Change Dem Volts", s=w839, f="Post Process") -> (s? t:f=w848:string)
          }
          frame "Post Process Raw Data File" {
          }
        }
      }
      frame "Change Dem Volts" {
        n384 = local read "WT Numbers"() -> (w883:string[])
        n385 = local read "All WTs"() -> (w904:dbl[][])
        n386 = for {
          N: 11 -> [_]
          tunnel: w907 -> [w966]
          tunnel: [w965] -> w880 mode=indexing
          tunnel: [w964] -> w895 mode=indexing
          tunnel: w904 -> [w962] mode=indexing
          tunnel: [w961] -> w878 mode=indexing
          tunnel: [w960] -> w889
          tunnel: w888 -> [w959]
          tunnel: w883 -> [w958] mode=indexing
          i -> [w967]
          n387 = Increment(x=w967) -> (x+1=w960:i32)
          n388 = Format Into String(format string=w966, w958) -> (resulting string=w964:string)  [unwired: 2 in, 1 out]
          n389 = Format Into String(format string=w959, w958) -> (resulting string=w965:string)  [unwired: 2 in, 1 out]
          n390 = Index Array(array=w962, index=0) -> (element=w961:dbl)
        }
        n391 = Build Array (concatenate)(w880, w895) -> (w906:string[])
        n392 = call "Get_Current_Scan_client.vi"("multipleChannels"=w906) -> ("Numerical Values"=w905:dbl[])  [unwired: 1 in, 3 out]
        n393 = Split 1D Array(array=w905, index=w889) -> (first subarray=w879:dbl[], second subarray=w871:dbl[])
        "Turbine Dem RPM" <- w879
        n394 = Divide(x=w879, y=w878) -> (x/y=w866:dbl[])
        n395 = In Range and Coerce(upper limit=1.005, x=w866, lower limit=0.995) -> (In Range?=w865:bool[])  [unwired: 1 out]
        n396 = for {
          tunnel: w865 -> [w911] mode=indexing
          tunnel: [w908] -> w864 mode=indexing
          n397 = Select(t=0.1 ("upper limit"), s=w911, f=0.4 ("upper limit")) -> (s? t:f=w908:dbl)
        }
        n398 = In Range and Coerce(upper limit=1.5, x=w866, lower limit=0.5) -> (coerced(x)=w874:dbl[], In Range?=w896:bool[])
        n399 = Decrement(x=w874) -> (x-1=w873:dbl[])
        n400 = Multiply(x=w873, y=w864) -> (x*y=w872:dbl[])
        n401 = Increment(x=w872) -> (x+1=w870:dbl[])
        n402 = Multiply(x=w871, y=w870) -> (x*y=w899:dbl[])
        n403 = In Range and Coerce(upper limit=12.0, x=w899, lower limit=0.0) -> (coerced(x)=w894:dbl[])  [unwired: 1 out]
        "Turbine Dem Voltage" <- w894
        n404 = for {
          shift-right: [w948] -> w892
          shift-left: string[] [] -> [w949]
          shift-right: [w946] -> w893
          shift-left: dbl[] [] -> [w947]
          tunnel: w896 -> [w943] mode=indexing
          tunnel: w895 -> [w945] mode=indexing
          tunnel: w894 -> [w944] mode=indexing
          tunnel: "Allow large changes?" -> [w941]
          n405 = Or(x=w941, y=w943) -> (x .or. y?=w942:bool)
          n406 = case shown="True" w942 {
            tunnel: w949 -> [w951 w957]
            tunnel: [w951 w956] -> w948
            tunnel: w947 -> [w950 w955]
            tunnel: [w950 w954] -> w946
            tunnel: w945 -> [_ w953]
            tunnel: w944 -> [_ w952]
            frame False {
            }
            frame True {
              n407 = Build Array (concatenate)(w957, w953) -> (w956:string[])
              n408 = Build Array (concatenate)(w955, w952) -> (w954:dbl[])
            }
          }
        }
        n409 = call "ASYNC_Adam_client.vi"("Values"=w893, "Channel Names"=w892) -> ()  [unwired: 1 in, 2 out]
        n410 = for {
          tunnel: w866 -> [w931] mode=indexing
          tunnel: w880 -> [w930] mode=indexing
          tunnel: w879 -> [w929] mode=indexing
          tunnel: w878 -> [w928] mode=indexing
          shift-right: [w925] -> w876
          shift-left: "" -> [w926]
          n411 = In Range and Coerce(upper limit=1.02, x=w931, lower limit=0.98) -> (In Range?=w927:bool)  [unwired: 1 out]
          n412 = case shown="False" w927 {
            tunnel: w930 -> [w939 _]
            tunnel: w929 -> [w938 _]
            tunnel: w928 -> [w937 _]
            tunnel: [w935 w940] -> w925
            tunnel: w926 -> [w934 w940]
            frame False {
              n413 = Format Into String(format string="%s=%.1f Measured is %.1f\n", initial string=w934, w939, w938, w937) -> (resulting string=w935:string)  [unwired: 1 in, 1 out]
            }
            frame True {
            }
          }
        }
        n414 = while {
          shift-right: [w916] -> _
          shift-left: _ -> [w915]
          shift-left: _ -> [w914]
          tunnel: w876 -> [w918]
          tunnel: [w913] -> w875
          stop <- TRUE stop-if-true
          n415 = Empty String/Path?(string/path=w918) -> (empty?=w917:bool)
          n416 = Not(x=w917) -> (.not. x?=w916:bool)
          n417 = Compound Arithmetic op=AND(w916, w915, w914) -> (w913:bool)
        }
        n418 = case shown="True" w875 {
          tunnel: w876 -> [_ w921]
          frame False {
          }
          frame True {
            n419 = Bundle By Name(cluster=errorcluster {"status"=FALSE, "code"=0, "source"=""} ("error in (no error)"), "source"=w921, "status"=TRUE) -> (w920:errorcluster)
            n420 = call "EnFlo_Error_Handler.vi"("error in (no error)"=w920, "Error Type"="Wind Turbine Speed Error", "Dialog Box (F)"=FALSE ("Dialog Box (T)")) -> ()  [unwired: 1 in, 2 out]
          }
        }
      }
      frame "Post Process" {
        n421 = Compound Arithmetic op=AND("Add Phase data to results file", w975) -> (w974:bool)
        n422 = case shown="True" w974 {
          tunnel: w973 -> [_ w981]
          tunnel: w969 -> [_ w980]
          frame False {
          }
          frame True {
            n423 = stacked-sequence {
              tunnel: w981 -> [w983 _]
              tunnel: w980 -> [_ w1009]
              frame #0 {
                n424 = local read "Channel to Phase lock"() -> (w990:i32[])
                n425 = property on="Channel to Phase lock" class="LstBox (strict)"() -> ("Item Names"=w989:string[])  [unwired: 2 in, 2 out]
                n426 = local read "Plug in titles"() -> (w984:string[])
                n427 = Divide(x=360, y=w983) -> (x/y=w986:dbl)
                n428 = Increment(x=w983) -> (x+1=w982:dbl)
                n429 = for {
                  tunnel: w989 -> [w1008]
                  tunnel: w990 -> [w1007] mode=indexing
                  tunnel: [w1006] -> w988 mode=indexing
                  n430 = Index Array(array=w1008, index=w1007) -> (element=w1006:string)
                }
                n431 = for {
                  tunnel: w988 -> [w997] mode=indexing
                  tunnel: w986 -> [w996]
                  shift-right: [w993] -> w985
                  shift-left: w984 -> [w995]
                  tunnel: w982 -> [w991]
                  n432 = for {
                    N: w991 -> [_]
                    tunnel: w997 -> [w1000]
                    tunnel: w996 -> [w1004]
                    tunnel: [w1002] -> w994 mode=indexing
                    tunnel: [w999] -> w992 mode=indexing
                    i -> [w1005]
                    n433 = Multiply(x=w1004, y=w1005) -> (x*y=w998:dbl)
                    n434 = Format Into String(format string="%s:Mean:%.1f Deg:%.1f", w1000, w998, w998) -> (resulting string=w1002:string)  [unwired: 2 in, 1 out]
                    n435 = Format Into String(format string="%s:Variance:%.1f Deg:%.1f", w1000, w998, w998) -> (resulting string=w999:string)  [unwired: 2 in, 1 out]
                  }
                  n436 = Build Array (concatenate)(w995, w994, w992) -> (w993:string[])
                }
                n437 = local write "Plug in titles"(w985) -> ()
              }
              frame #1 {
                n438 = local read "Plug in values"() -> (w1011:string[])
                n439 = for {
                  tunnel: w1009 -> [w1014] mode=indexing
                  shift-right: [w1017] -> w1010
                  shift-left: w1011 -> [w1018]
                  n440 = Unbundle(w1014) -> (w1012:dbl[], w1013:dbl[])
                  n441 = for {
                    tunnel: w1012 -> [w1021] mode=indexing
                    tunnel: [w1022] -> w1016 mode=indexing
                    tunnel: w1013 -> [w1019] mode=indexing
                    tunnel: [w1020] -> w1015 mode=indexing
                    n442 = call "Number_2_string.vi"("number"=w1021) -> ("String"=w1022:string)  [unwired: 1 in]
                    n443 = call "Number_2_string.vi"("number"=w1019) -> ("String"=w1020:string)  [unwired: 1 in]
                  }
                  n444 = Build Array (concatenate)(w1018, w1016, w1015) -> (w1017:string[])
                }
                n445 = local write "Plug in values"(w1010) -> ()
              }
            }
          }
        }
        n446 = Compound Arithmetic op=AND("Save Phase averaged Profiles", w975) -> (w977:bool)
      }
      frame "Check Folder Name" {
        n447 = File/Directory Info(path="Output Directory") -> (error out=w1032:errorcluster)  [unwired: 1 in, 6 out]
        n448 = Empty String/Path?(string/path="Output Directory") -> (empty?=w1034:bool)
        n449 = Unbundle By Name(w1032) -> ("status"=w1033:bool)
        n450 = Or(x=w1034, y=w1033) -> (x .or. y?=w1035:bool)
        n451 = case shown="True" w1035 {
          tunnel: [w1038 w1044] -> w1028
          tunnel: "Output Directory" -> [w1038 w1042]
          tunnel: [FALSE ("cancelled") w1039] -> w1030
          frame False {
          }
          frame True {
            n452 = Strip Path(path=w1042) -> (stripped path=w1041:path, name=w1040:string)
            n453 = File Dialog(7:"Please Select a new or existing Results folder" ("prompt"), 9:w1040, 11:w1041) -> (1:w1039:bool, 3:w1044:path)  [unwired: 1 in, 5 out]
          }
        }
        n454 = local write "Output Directory"(w1028) -> ()
        n455 = Not(x=w1030) -> (.not. x?=w1029:bool)
      }
      frame "Save Phase locked data" {
        n456 = global read "Meas_global.vi" "Raw data file"() -> (w1052:path)
        n457 = stacked-sequence {
          seq-local: [_ w1081 _ _] -> [_ _ _ w1139]
          seq-local: [w1059 _ _ _] -> [_ _ _ w1140]
          seq-local: [_ _ w1096 _] -> [_ _ _ w1138]
          seq-local: [w1054 _ _ _] -> [_ _ w1095 _]
          tunnel: w1052 -> [w1058 _ _ w1144]
          tunnel: w1048 -> [w1057 _ _ _]
          tunnel: w1047 -> [_ _ w1094 _]
          frame #0 {
            w1060 = "\r\n"
            n458 = for {
              tunnel: w1057 -> [w1065] mode=indexing
              tunnel: [w1063] -> w1056 mode=indexing
              tunnel: [w1064] -> w1055 mode=indexing
              n459 = Unbundle(w1065) -> (w1063:dbl[], w1064:dbl[])
            }
            n460 = call "Read_RD_Ch_header.vi"("Raw data file"=w1058) -> ("Ch string"=w1062:string)  [unwired: 3 out]
            n461 = Concatenate Strings(w1060, "*****This is a many rows per single point file*****", w1060, w1062) -> (w1059:string)
            n462 = Build Array (concatenate)(w1056, w1055) -> (w1054:dbl[][])
          }
          frame #1 {
            w1067 = "\r\n"
            n463 = local read "Channel to Phase lock"() -> (w1083:i32[])
            n464 = property on="Channel to Phase lock" class="LstBox (strict)"() -> ("Item Names"=w1082:string[])  [unwired: 2 in, 2 out]
            n465 = Initialize Array("", 10) -> (w1084:string[])
            n466 = call "Asterisk_header.vi"("Channel names"=w1084) -> ("Header string"=w1066:string)
            n467 = for {
              tunnel: w1083 -> [w1092] mode=indexing
              tunnel: w1082 -> [w1091]
              tunnel: [w1090] -> w1079 mode=indexing
              tunnel: ["Mean" ("format string")] -> w1077 mode=indexing
              tunnel: ["Variance" ("format string")] -> w1076 mode=indexing
              tunnel: [""] -> w1074 mode=indexing
              n468 = Index Array(array=w1091, index=w1092) -> (element=w1090:string)
            }
            n469 = Build Array (concatenate)("Rotor", w1079, w1079) -> (w1073:string[])
            n470 = Build Array (concatenate)("Angle", w1077, w1076) -> (w1072:string[])
            n471 = Build Array (concatenate)("(deg)", w1074, w1074) -> (w1071:string[])
            n472 = Build Array(w1073, w1072, w1071) -> (w1070:string[][])
            n473 = Array To Spreadsheet String(array=w1070, 3:"%s" ("format string")) -> (spreadsheet string=w1068:string)  [unwired: 1 out]
            n474 = Concatenate Strings(w1067, w1066, w1068, w1067) -> (w1081:string)
          }
          frame #2 {
            n475 = Array Size(array=w1095) -> (size(s)=w1097:i32[])
            n476 = Index Array(array=w1097, index=0) -> (element=w1102:i32)
            n477 = Index Array(array=w1097, index=1) -> (element=w1098:i32)
            n478 = Decrement(x=w1102) -> (x-1=w1103:i32)
            n479 = for {
              N: w1098 -> [_]
              shift-right: [w1119] -> w1096
              shift-left: "" -> [w1114]
              tunnel: "Separation Character" -> [w1111]
              tunnel: w1095 -> [w1117]
              tunnel: w1103 -> [w1113]
              tunnel: w1094 -> [w1108]
              tunnel: [w1104] -> _ mode=indexing
              i -> [w1110]
              n480 = Divide(x=w1108, y=2.0) -> (x/y=w1106:dbl)
              n481 = Multiply(x=w1110, y=w1108) -> (x*y=w1105:dbl)
              n482 = Index Array(array=w1117, index (col)=w1110) -> (element=w1116:dbl[])  [unwired: 1 in]
              n483 = Add(x=w1105, y=w1106) -> (x+y=w1104:dbl)
              n484 = call "Number_2_string.vi"("number"=w1104) -> ("String"=w1109:string)  [unwired: 1 in]
              n485 = Concatenate Strings(w1109, w1111) -> (w1112:string)
              n486 = for {
                shift-right: [w1127] -> w1115
                shift-left: w1112 -> [w1128]
                tunnel: w1111 -> [w1126]
                tunnel: w1116 -> [w1122] mode=indexing
                tunnel: w1113 -> [w1124]
                i -> [w1125]
                n487 = Equal?(x=w1125, y=w1124) -> (x = y?=w1123:bool)
                n488 = call "Number_2_string.vi"("precision"="Precision", "number"=w1122) -> ("String"=w1121:string)
                n489 = case shown="False" w1123 {
                  tunnel: w1128 -> [w1132 w1135]
                  tunnel: w1121 -> [w1131 w1134]
                  tunnel: [w1130 w1133] -> w1127
                  tunnel: w1126 -> [w1129 _]
                  frame False {
                    n490 = Concatenate Strings(w1132, w1131, w1129) -> (w1130:string)
                  }
                  frame True {
                    n491 = Concatenate Strings(w1135, w1134) -> (w1133:string)
                  }
                }
              }
              n492 = Concatenate Strings(w1114, w1115, "\r\n") -> (w1119:string)
            }
          }
          frame #3 {
            w1136 = FALSE  # append to file? (new file:F)
            n493 = Strip Path(path=w1144) -> (name=w1142:string)  [unwired: 1 out]
            n494 = local read "Output Directory"() -> (w1143:path)
            n495 = Build Path(base path=w1143, name or relative path=w1142) -> (appended path=w1141:path)
            n496 = Concatenate Strings(w1140, w1139, w1138) -> (w1137:string)
            n497 = call "Write_File_Simple.vi"("append to file? (new file:F)"=w1136, "character string"=w1137, "file path"=w1141) -> ()  [unwired: 2 out]
          }
        }
      }
    }
  }
